vi "Main.vi"() -> ()   [LabVIEW 2020]
doc: "This Continuous Measurement sample project is based on the Queued Message Handler template.\n\nThe Event Handling Loop generates messages based on user interface actions.\n\nThe Message Handling Loop processes messages generated by the Event Handling Loop, or by other messages. There are also Acquisition and Logging message handling loop subVIs, and a chart updating loop."
uses:
  controls/UI Data.ctl
  Modbus/Modbus All Data.ctl
  Modbus/Modbus PLC Data All.ctl
  Modbus/Modbus FVIR Control.ctl
  Modbus/Modbus LDO Control.ctl
  WritingDataFile/Data to Save.ctl
  Modbus/Modbus Gas Meter Data.ctl
  Drivers/Alicat LabVIEW Drivers 2v1/Sub-VIs/Data Cluster.ctl
  Drivers/Alicat LabVIEW Drivers 2v1/Sub-VIs/Units of Measure.ctl
  Drivers/Inficon Transmitter/Type Definitions/Inficon Data.ctl
  support/Event Booleans.ctl
  support/Message Queue/Enqueue Message (Single).vi
  <vilib>/Utility/error.llb/Error Cluster From Error Code.vi
  <vilib>/ErrorRing/Error Ring.xnode
  support/User Event - Stop/User Event - Stop.lvlib
  support/Message Queue/Message Queue.lvlib
  Modbus/Modbus.lvlib
  ReadingDataFile/ReadingDataFile.lvlib
  WritingDataFile/WritingDataFile.lvlib
panel:
  in  "Start Auto GPM Gallons":dbl=5.0 format="%#_13g"
  in  "Debug":bool
  out "Message Loop":string[](array[string])
  out "Event Loop":i32
  out "UI Message Loop":i32
  in  "Tab Control":enum32{"FVIR", "LDO", "Administrator"}(tab)
  out "Actuator spill can is going to Work Pos - FVIR":bool
  out "Actuator spill can is going to Home Pos - FVIR":bool
  out "Actuator mannequin is going to Work Pos - FVIR":bool
  out "Actuator mannequin is going to Home Pos - FVIR":bool
  out "Error - FVIR":bool caption="Error"
  out "Status for error - FVIR":string caption="Error status for FVIR"
  in  "Move mannequin - Go to Work Pos":bool
  in  "Move mannequin - Go to Home Pos":bool
  in  "Spill can - Go to Work Pos":bool
  in  "Spill can - Go to Home Pos":bool
  out "Start recording data - FVIR":bool
  out "Test chamber is in sequence - FVIR":bool
  out "Can is spilling - FVIR":bool
  out "Mannequin is moving - FVIR":bool
  in  "Select test case":i32(listbox)
  in  "Stop Test Case FVIR":bool
  in  "Start Test Case FVIR":bool
  in  "Water Outlet Valve Close FVIR":bool
  in  "Water Outlet Valve Open FVIR":bool
  in  "Gas Solenoid Valve Close FVIR":bool
  in  "Gas Solenoid Valve Open FVIR":bool
  in  "Water Inlet Valve Close FVIR":bool
  in  "Water Inlet Valve Open FVIR":bool
  in  "Water Flow Intellifaucet DRK375 Close FVIR":bool
  in  "Water Flow Intellifaucet DRK375 Open FVIR":bool
  out "Temperatures - FVIR":string[][](array[string])
  out "Sensors - FVIR":string[][](array[string])
  in  "Water Outlet Flow Proportional Valve EPV-312B Close FVIR":bool
  in  "Water Outlet Flow Proportional Valve EPV-312B Open FVIR":bool
  out "Water Outlet Flow Proportional - FVIR":bool
  out "Water flow DRK375 is open - FVIR":bool
  out "Gas Solenoid Valuce - FVIR":bool
  out "Water Inlet Valve - FVIR":bool
  out "Water Outlet Valve - FVIR":bool
  out "General status for FVIR":string
  out "Higher than 1.8% butane":bool
  in  "Start":bool
  in  "Stop":bool
  in  "Path to local logfile":path=path "C:/Users/christian.hansen/Desktop/GE Appliance - FVIR/GEA_Labview_FVIR/CH1234dummy.LOG"
  in  "Reset Flow Meter":bool
  in  "Blower OFF":bool
  in  "Blower ON":bool
  in  "Conveyor OFF":bool
  in  "Conveyor ON":bool
  out "Blower":bool
  out "Conveyor":bool
  in  "Gas Meter Tare Total":bool
  in  "Gas Meter Tare Rate":bool
  out "Data":string[][](array[string])
  in  "Proportioning Valve":dbl(slide) max=100.0 scale=0.0..100.0
  in  "Valve % Open":dbl(slide)=15.0 min=15.0 max=100.0 scale=15.0..100.0
  in  "Temp (°F)":dbl(slide)=32.0 min=32.0 max=203.0 scale=32.0..200.0
  in  "Water Flow Intellifaucet DRK375 Open LDO":bool
  in  "Water Flow Intellifaucet DRK375 Close LDO":bool
  out "Rotary Actuator (ON/OFF)":bool
  out "Oil spray 1.33cc/min":bool
  out "Oil spray 1.1cc/min":bool
  out "Oil spray 0.8cc/min":bool
  out "Burner":bool
  out "Start recording data - LDO":bool
  out "Test chamber is in sequence":bool
  in  "Stop Test Case LDO":bool
  in  "Start Test Case LDO":bool
  in  "Water Outlet Valve Close LDO":bool
  in  "Water Outlet Valve Open LDO":bool
  in  "Water Inlet Valve Close LDO":bool
  in  "Water Inlet Valve Open LDO":bool
  in  "Gas Solenoid Valve Close LDO":bool
  in  "Gas Solenoid Valve Open LDO":bool
  in  "Oil Spray 0.8 cc/min Close":bool
  in  "Oil Spray 0.8 cc/min Open":bool
  in  "Oil Spray 1.1 cc/min Close":bool
  in  "Oil Spray 1.1 cc/min Open":bool
  in  "Oil Spray 1.33 cc/min Close":bool
  in  "Oil Spray 1.33 cc/min Open":bool
  in  "Heater OFF":bool
  in  "Heater ON":bool
  out "Water Outlet Flow Proportional":bool
  out "Intellifaucet Start":bool
  out "Gas Solenoid Valve":bool
  out "Water Inlet Valve":bool
  out "Water Outlet Valve":bool
  in  "Temp (°F) - Automatic Mode":dbl=70.0 min=32.0 max=203.0
  in  "Valve % Open - Automatic Mode":dbl=50.0 min=15.0 max=100.0
  in  "Precondition Purge Gallons":u16=200 caption="Precondition Purge Time (Sec)"
  in  "Pilot Rate (BTU/hr)":dbl=600.0
  out "FVIR PLC lifebit":bool
  out "Labview lifebit":bool
  in  "Send parameters to PLC LDO":bool
  in  "Burner cycle 1 to 10 - Duty cycle ON (default 55 min.)":u16=55 caption="Burner cycle 1 to 10 - Duty cycle ON"
  in  "Burner cycle 1 to 10 - Duty cycle OFF (default 5 min.)":u16=5 caption="Burner cycle 1 to 10 - Duty cycle OFF"
  in  "Burner cycle 11 to 12 - Duty cycle ON (default 235 min.)":u16=235 caption="Burner cycle 11 to 12 - Duty cycle ON"
  in  "Burner cycle 11 to 12 - Duty cycle OFF (default 5 min.)":u16=5 caption="Burner cycle 11 to 12 - Duty cycle OFF"
  in  "Burner cycle 13 to end - Duty cycle ON (default 55 min.)":u16=55 caption="Burner cycle 13 to end - Duty cycle ON"
  in  "Burner cycle 13 to end - Duty cycle OFF (default 5 min.)":u16=5 caption="Burner cycle 13 to end - Duty cycle OFF"
  in  "Oil 1st sequence ON (default 5 min.)":u16=5 caption="Oil 1st sequence ON"
  in  "Oil 1st sequence OFF (default 5 min.)":u16=25 caption="Oil 1st sequence OFF"
  in  "All subsequent sequence ON (default 3 min.)":u16=3 caption="All subsequent sequence ON"
  in  "All subsequent sequence OFF (default 27 min.)":u16=27 caption="All subsequent sequence OFF"
  in  "Oil spray preconditioning period ON (default 10 min.)":u16=10 caption="Oil spray preconditioning period ON"
  in  "Oil spray preconditioning period OFF  (default 20 min.)":u16=20 caption="Oil spray preconditioning period OFF"
  out "General status for LDO":string
  out "Status for error - LDO":string caption="Error status for LDO"
  out "Error - LDO":bool caption="Error"
  in  "PLC IP address":string="10.2.0.11"
  in  "Inficon IP Address":string="192.168.1.32"
  in  "Ultramat 23":refnum<visa-resource-name>="ULTRAMAT"
  in  "Alicat VISA":refnum<visa-resource-name>="ALICAT_40SLPM"
  in  "Send parameters to PLC FVIR":bool
  in  "Time Pause Between Next Mannequin Sequence":u16=60
  in  "Water Flow Intellifaucet DRK375":u16=15
  in  "Water Temperature Intellifaucet DRK375":u16=70
  in  "Water Outlet Proportional Valve EPV-312B":u16=3
  in  "Number of Mannequin Movement":u16=3
  in  "Time Delay of Change direction of Mannequin Actuators":u16=1000
  # "FVIR and LDO:Swap the data, i.e. 28-10-2021 --> 2021-10-28. --> Lets test this first to see the currents PC timeformat. \nAll data is in the file now. Also the status of LEDs and what Labview is sending --> A lot of redundant info here. What from \nLabview --> PLC should be recorded?"
  # "FVIR: Missing implementation: Getting the glas flow rate, SQRH. CO, CO2 and O2 from the VI's from GEA"
  # "FVIR"
  # "Main control"
  # "Actuator spill can is going to Work Pos"
  # "Actuator spill can is going to Home Pos"
  # "Actuator mannequin is going to Work Pos"
  # "Actuator mannequin is going to Home Pos"
  # "Automatic mode"
  # "Start recording FVIR data"
  # "Test chamber is in sequence"
  # "Can is spilling"
  # "Mannequin is moving"
  # "Water Outlet Valve"
  # "Gas Solenoid Valve"
  # "Water Inlet Valve"
  # "Water Flow Intellifaucet DRK375"
  # "Water Outlet Flow Proportional EPV-312B"
  # "Water Outlet Flow Proportional is open"
  # "Water flow DRK375 is open"
  # "Gas Solenoid is open"
  # "Water Inlet is open"
  # "Water Outlet is open"
  # "Status of valves"
  # "Manual mode"
  # "Temperature from textfile - 4 channels"
  # "Status of actuators"
  # "Values from FVIR sensors"
  # "Status of chamber"
  # "Main control"
  # "Manual mode"
  # "Rotary Actuator"
  # "Status of devices"
  # "Status of chamber"
  # "Status of valves"
  # "Water Flow Intellifaucet DRK375"
  # "Water Flow Meter"
  # "Blower Control"
  # "Conveyor Control"
  # "Gas Meter"
  # "Automatic mode"
  # "Start and stop LDO test"
  # "Water Outlet Valve"
  # "Water Inlet Valve"
  # "Gas Solenoid Valve"
  # "Oil spray at 0.8 cc/min"
  # "Oil spray at 1.1 cc/min"
  # "Oil spray at 1.33 cc/min"
  # "LDO Parameters -"
  # "Changing parameters to PLC"
  # "FVIR Changing parameters to PLC"
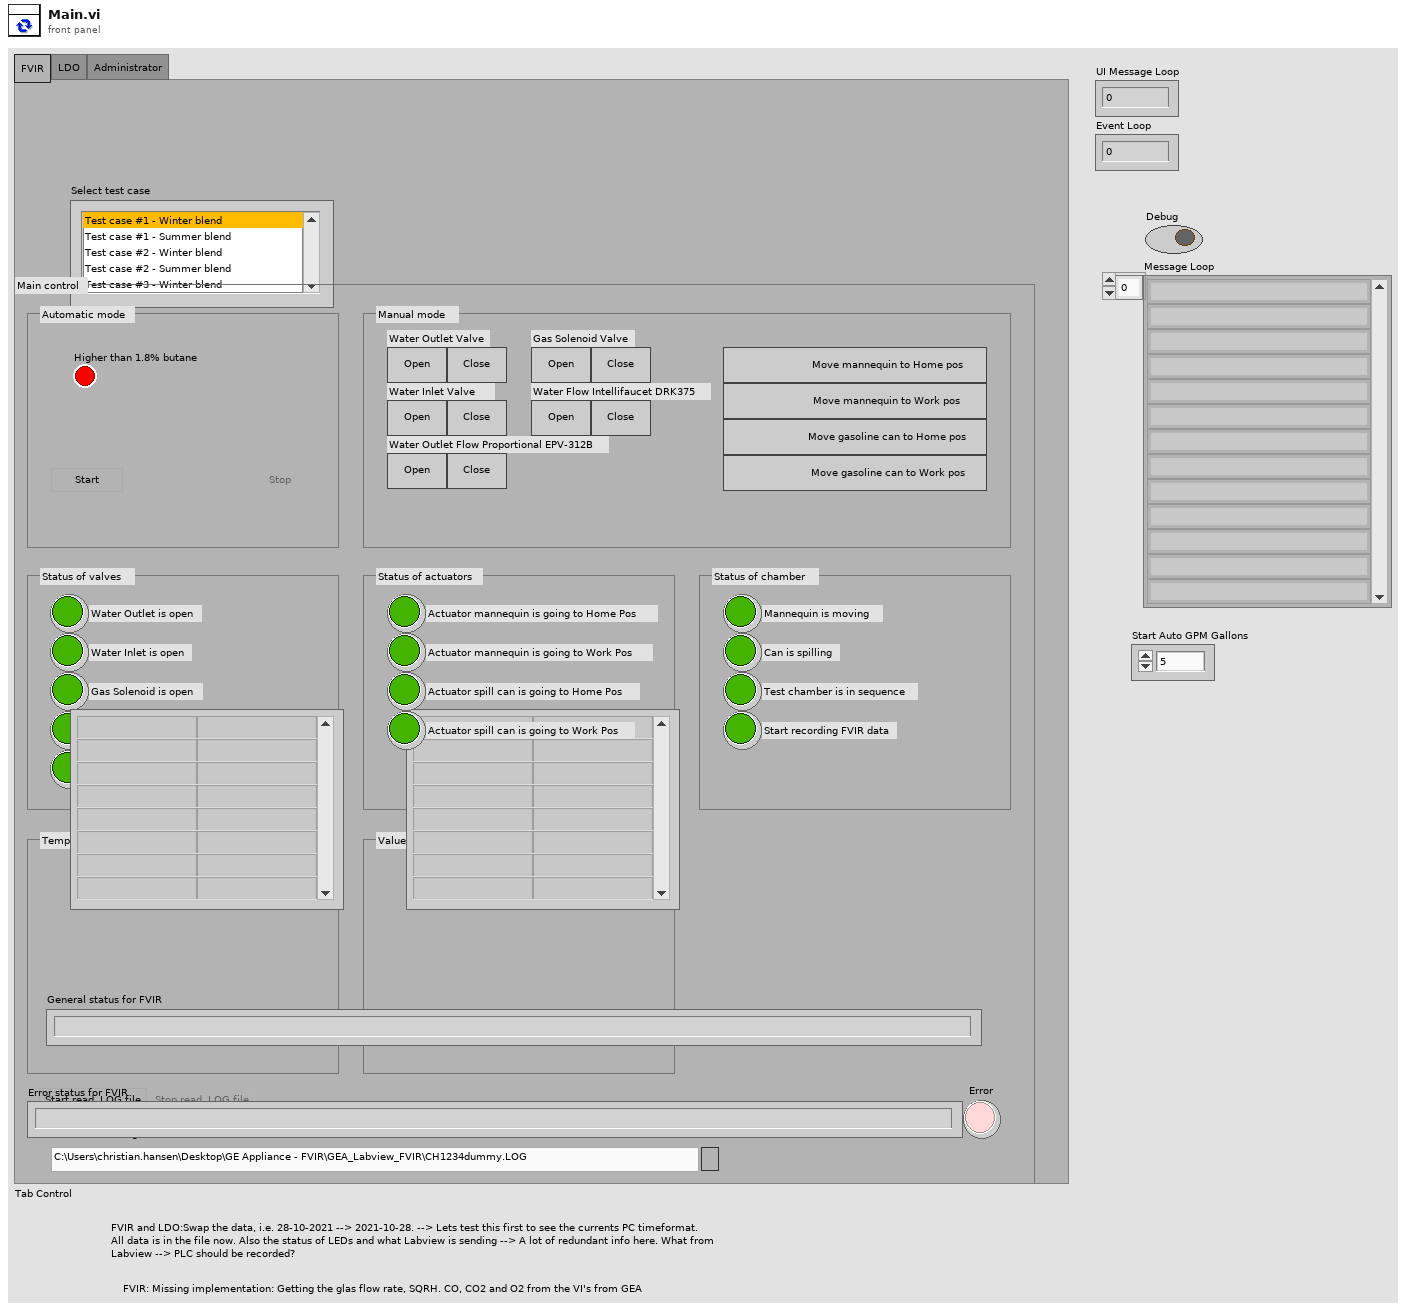
[diagram p1: front panel]
types:
  T1 = typedef "Event Booleans.ctl" = cluster{"Burner ON":bool, "0.8 ml Bool":bool, "1.1 Bool":bool, "1.33 Bool":bool, "Start recording data-LDO":bool}
  T2 = typedef "Modbus All Data.ctl" = cluster{"PLC Data Out":T3, "Gas Data":T7, "Inficon Data Input":T10, "Ultramat 23":string[][]}
  T3 = typedef "Modbus PLC Data All.ctl" = cluster{"FVIR Data Input":T4, "LDO Control Input":T5, "PLC Input Registers":i16[], "Data to Save":T6}
  T4 = typedef "Modbus FVIR Control.ctl" = cluster{"Spare 15":bool, "Spare 14":bool, "Actuator mannequin is going to Work Pos - FVIR":bool, "Actuator mannequin is going to Home Pos - FVIR":bool, "Test chamber is in sequence - FVIR ":bool, "Water flow DRK375 is open - FVIR":bool, "Gas Solenoid Valve - FVIR":bool, "Water Inlet Valve - FVIR":bool, "Water Outlet Flow Proportional - FVIR":bool, "Start recording data - FVIR":bool, "Actuator spill can is going to Work Pos - FVIR":bool, "Actuator spill can is going to Home Pos - FVIR":bool, "Water Outlet Valve - FVIR":bool, "Can is spilling - FVIR":bool, "Mannequin is moving - FVIR":bool, "FVIR PLC lifebit":bool, "Status for Error - FVIR":string, "Error-FVIR":bool, "Sensors -FVIR":string[][]}
  T5 = typedef "Modbus LDO Control.ctl" = cluster{"LDO PLC Life Bit":bool, "Start recording data - LDO":bool, "Spare 1":bool, "Water Outlet Valve - LDO":bool, "Water Inlet Valve - LDO":bool, "Gas Solenoid Valve - LDO":bool, "Water flow DRK375 is open - LDO":bool, "Test chamber is in sequence - LDO":bool, "Oil spray 0.8cc/min - LDO":bool, "Oil spray 1.1cc/min - LDO":bool, "Oil spray 1.33cc/min - LDO":bool, "Rotary Actuator (ON/OFF) - LDO":bool, "Water Outlet Flow Proportional - LDO":bool, "Conveyor ON/OFF":bool, "Blower ON/OFF":bool, "Spare 4":bool, "Status for error - LDO":string, "Error - LDO":bool, "Sensor Data":string[][], "Thermal Efficiency Rate (GPM)":dbl, "Thermal Efficiency":dbl, "Totalized Flow (Gallons)":dbl, "Counter of oil injections 1.33 cc/min":u16, "Counter of burner cycle":u16, "Counter of oil injections 1.1 cc/min":u16, "Counter of oil injections 0.8 cc/min":u16, "Previous Totalizer (Gallons)":dbl, "Gallon Adder Input":dbl}
  T6 = typedef "Data to Save.ctl" = cluster{"LDO Full Data":string[][], "FVIR Full Data":string[][], "Test Case - FVIR":string, "Test Case - LDO":string}
  T7 = typedef "Modbus Gas Meter Data.ctl" = cluster{"Data Cluster":T8, "Units of Measure Input":T9, "Header Array":string[]}
  T8 = typedef "Data Cluster.ctl" = cluster{"Absolute Pressure":dbl, "Gauge/Diff. Pressure":dbl, "Barometric Pressure":dbl, "Temperature":dbl, "Volumetric Flow":dbl, "Mass Flow":dbl, "Setpoint":dbl, "Valve Drive":dbl, "Totalizer":dbl, "[hr]":dbl, "[min]":dbl, "[sec]":dbl, "Totalizer Average Flow":dbl, "Totalizer Peak Flow":dbl, "Gas selected":string}
  T9 = typedef "Units of Measure.ctl" = cluster{"Abs. Pressure":string, "Gauge/Diff. Press.":string, "Barometric Press.":string, "Temperature":string, "Volume":string, "Mass":string, "Setpoint":string, "Valve Drive":string, "Totalizer":string, "Tot. Timer":string, "Tot. Avg. Flow":string, "Tot. Peak Flow":string}
  T10 = typedef "Inficon Data.ctl" = cluster{"Gross Heating Value, Vol (Real, Dry)":dbl, "Nitrogen Component Normalized Mole % (Dry)":dbl, "Methane Component Normalized Mole % (Dry)":dbl, "Carbon Dioxide Component Normalized Mole % (Dry)":dbl, "Ethane Component Normalized Mole % (Dry)":dbl, "Propane Component Normalized Mole % (Dry)":dbl, "i-Pentane Component Normalized Mole % (Dry)":dbl, "i-Butane Component Normalized Mole % (Dry)":dbl, "n-Butane Component Normalized Mole % (Dry)":dbl, "n-Pentane Component Normalized Mole % (Dry)":dbl, "Hexane Component Normalized Mole % (Dry)":dbl, "Heptane Component Normalized Mole % (Dry)":dbl, "Gross Wobbe Index, Real(Dry)":dbl, "Relative Density, Real(Dry)":dbl, "Propylene Component Normalized Mole % (Dry)":dbl, "C4 Olefins Component Normalized Mole % (Dry)":dbl, "Water Component Normalized Mole % (Dry)":dbl}
  T11 = typedef "UI Data.ctl" = cluster{"Start Ref":refnum<vi>, "Stop Ref":refnum<vi>, "Exit Ref":refnum<vi>, "Status Ref":refnum<vi>, "Connect Ref":refnum<vi>, "Disconnect Ref":refnum<vi>, "Spill can Home pos Ref":refnum<vi>, "Spill can Work pos Ref":refnum<vi>, "Move Mannequin Home pos Ref":refnum<vi>, "Move Mannequin Work pos Ref":refnum<vi>, "Start test case FVIR Ref":refnum<vi>, "Water Outlet Valve Open FVIR Ref":refnum<vi>, "Water Inlet Valve Open FVIR Ref":refnum<vi>, "Gas Solenoid Valve Open FVIR Ref":refnum<vi>, "Water Flow Open FVIR Ref":refnum<vi>, "Listbox Ref":refnum<vi>, "Stop test case FVIR Ref":refnum<vi>, "Water Outlet Valve Close FVIR Ref":refnum<vi>, "Water Inlet Valve Close FVIR Ref":refnum<vi>, "Gas Solenoid Valve Close FVIR Ref":refnum<vi>, "Water Flow Close FVIR Ref":refnum<vi>, "Send Param to PLC FVIR Ref":refnum<vi>, "Water Flow Prop Open FVIR Ref":refnum<vi>, "Water Flow Prop Close FVIR Ref":refnum<vi>, "Start test case LDO Ref":refnum<vi>, "Stop test case LDO Ref":refnum<vi>, "Water Outlet Valve Open LDO Ref":refnum<vi>, "Water Outlet Valve Close LDO Ref":refnum<vi>, "Water Inlet Valve Open LDO Ref":refnum<vi>, "Water Inlet Valve Close LDO Ref":refnum<vi>, "Gas Solenoid Valve Open LDO Ref":refnum<vi>, "Gas Solenoid Valve Close LDO Ref":refnum<vi>, "Water Flow Open LDO Ref":refnum<vi>, "Water Flow Close LDO Ref":refnum<vi>, "Water Flow Prop Open LDO Ref":refnum<vi>, "Water Flow Prop Close LDO Ref":refnum<vi>, "Oil spray 0.8cc/min Open Ref":refnum<vi>, "Oil spray 0.8cc/min Close Ref":refnum<vi>, "Oil spray 1.1cc/min Open Ref":refnum<vi>, "Oil spray 1.1cc/min Close Ref":refnum<vi>, "Oil spray 1.33cc/min Open Ref":refnum<vi>, "Oil spray 1.33cc/min Close Ref":refnum<vi>, "Heater ON Ref":refnum<vi>, "Heater OFF Ref":refnum<vi>, "Send Param to PLC LDO Ref":refnum<vi>}
  T12 = typedef "Message Queue.lvlib/All Message Queues.ctl" = cluster{"UI":refnum<queue>, "Modbus":refnum<queue>, "Watchdog":refnum<queue>, "ReadDataFile":refnum<queue>, "DataScanning":refnum<queue>, "WriteDataFile":refnum<queue>, "WatchdogWriteFile":refnum<queue>, "OilMachine":refnum<queue>, "Alicat_GasMeter":refnum<queue>, "Inficon":refnum<queue>, "Ultramat 23":refnum<queue>}
  T13 = enum8{"Enabled", "Disabled", "Disabled and Grayed Out"}
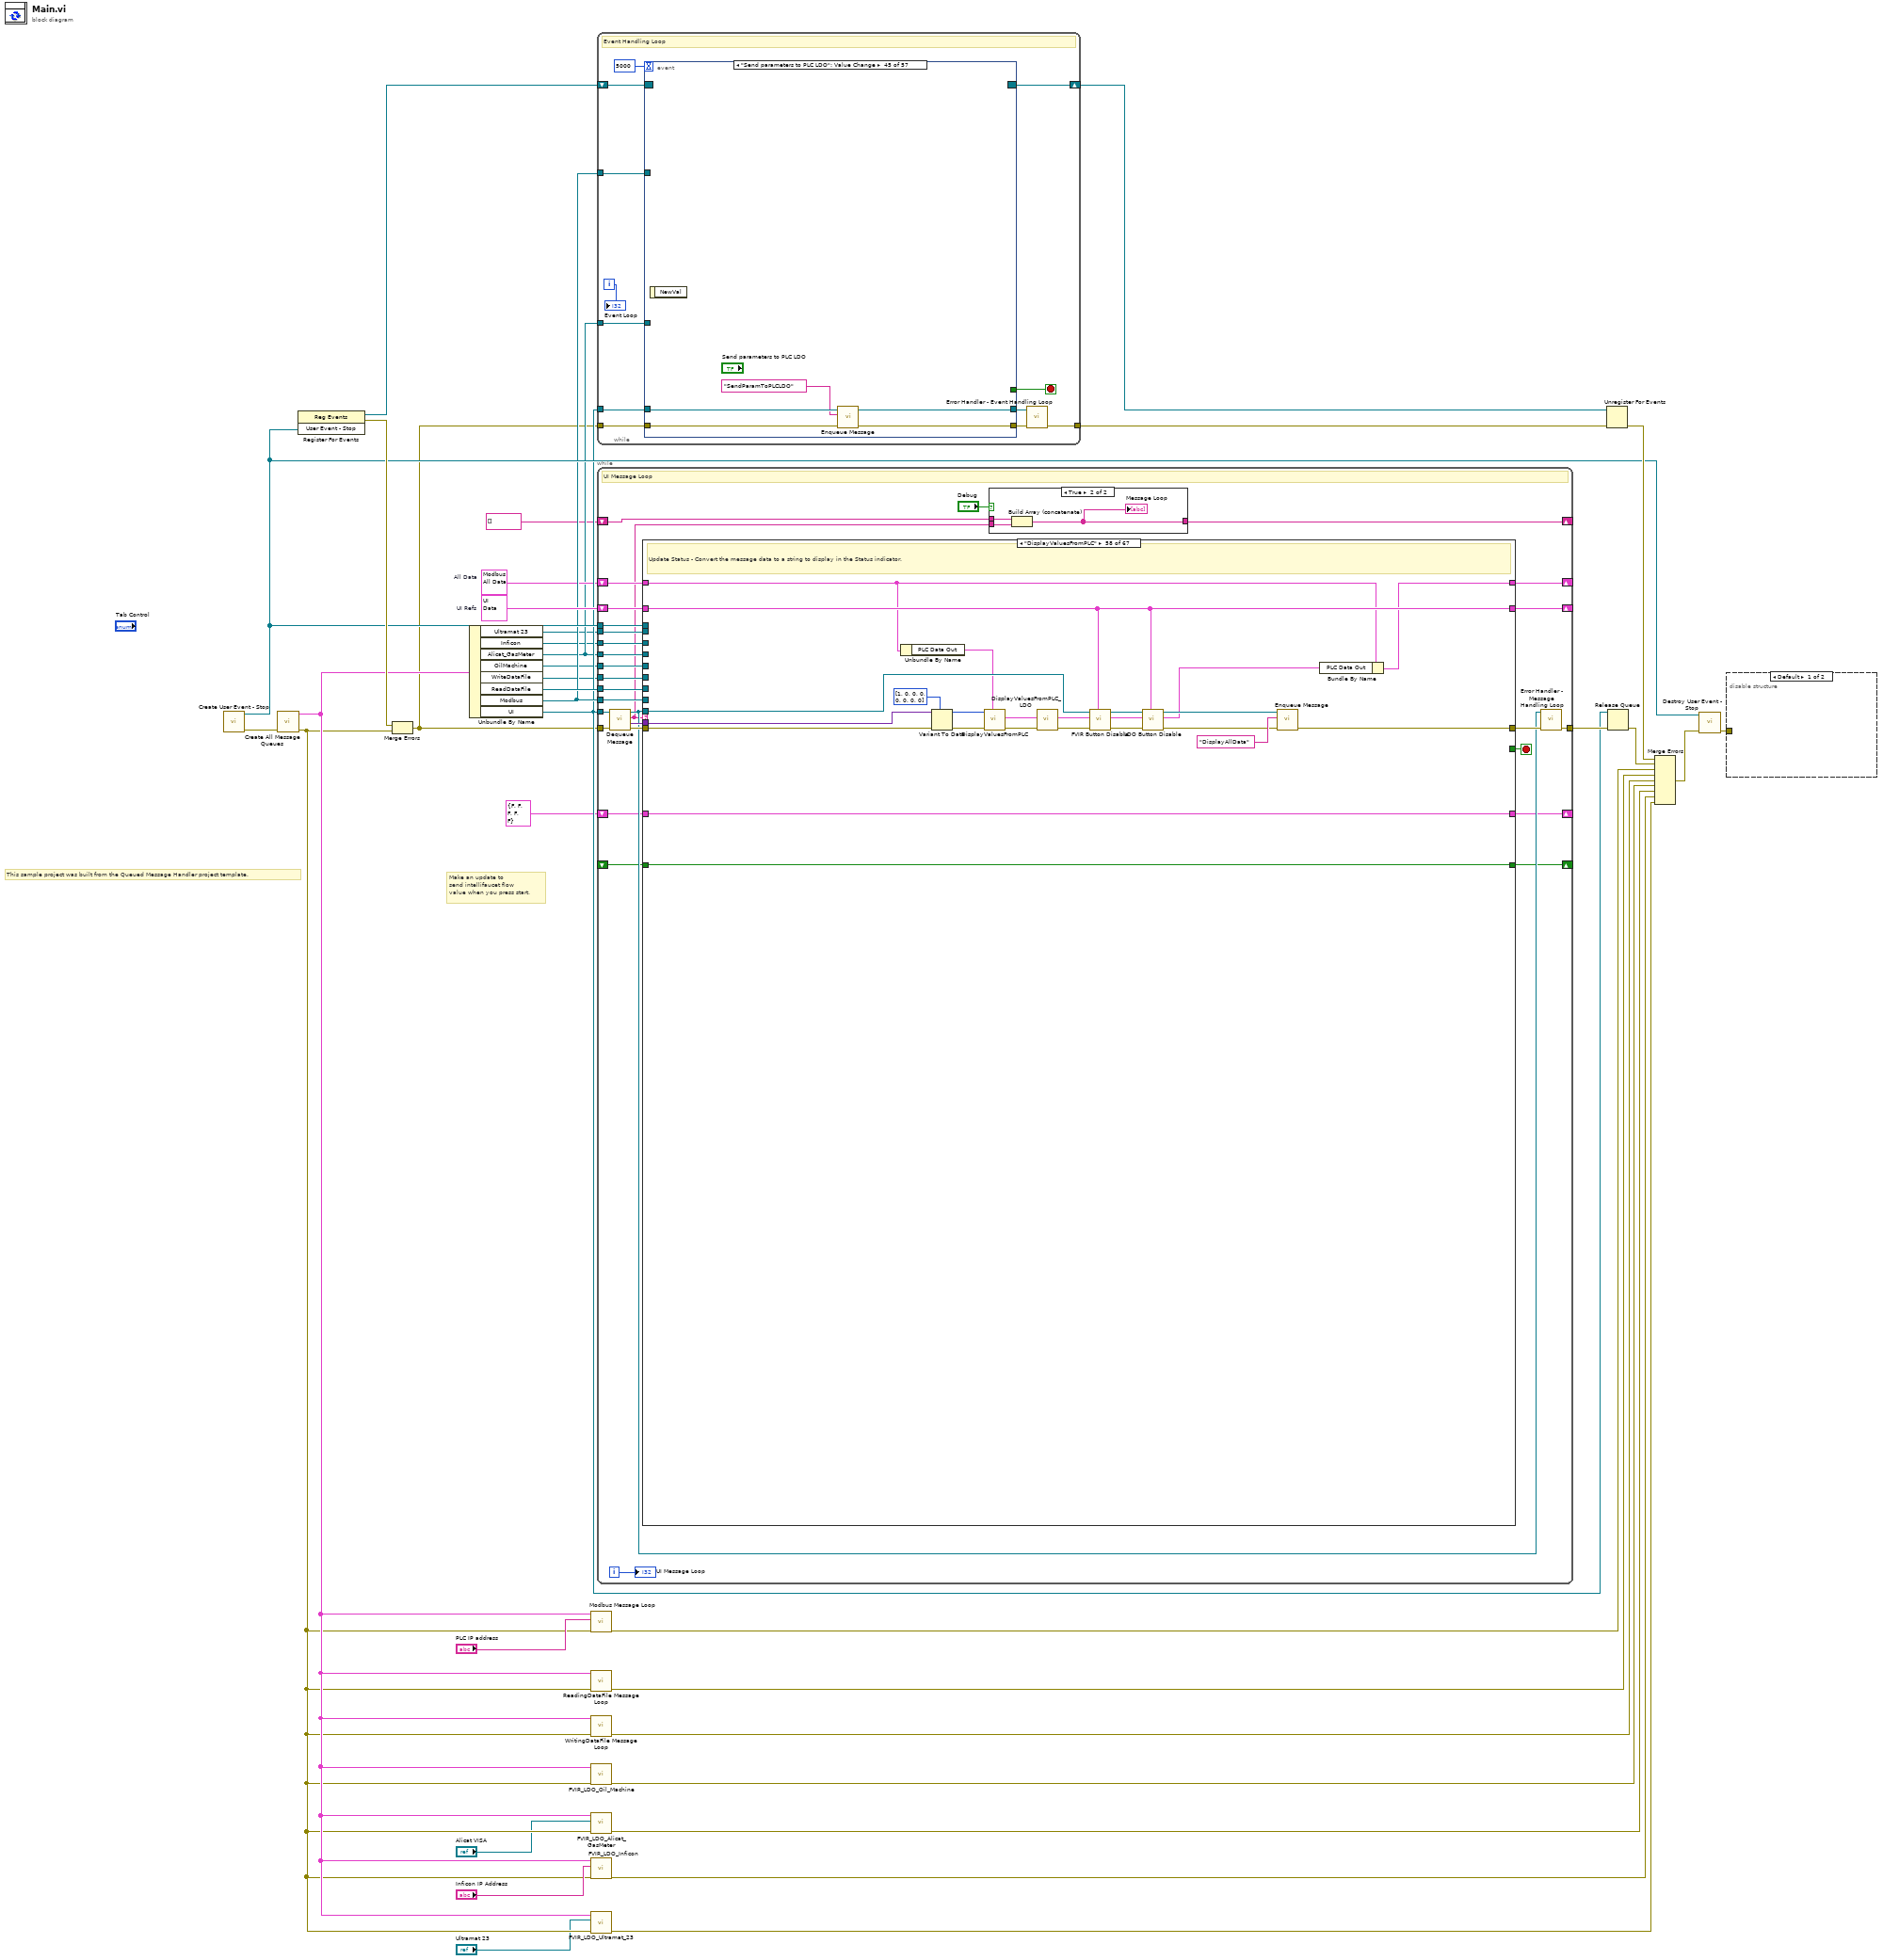
[diagram p0: block diagram]
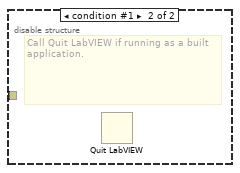
[diagram p2: hidden frame]
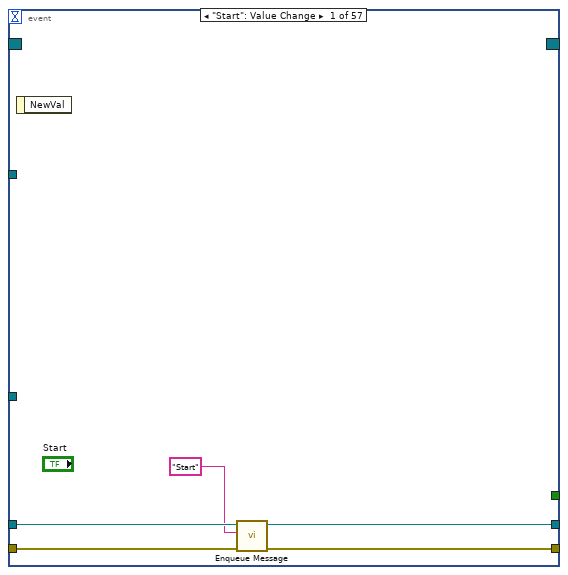
[diagram p3: hidden frame]
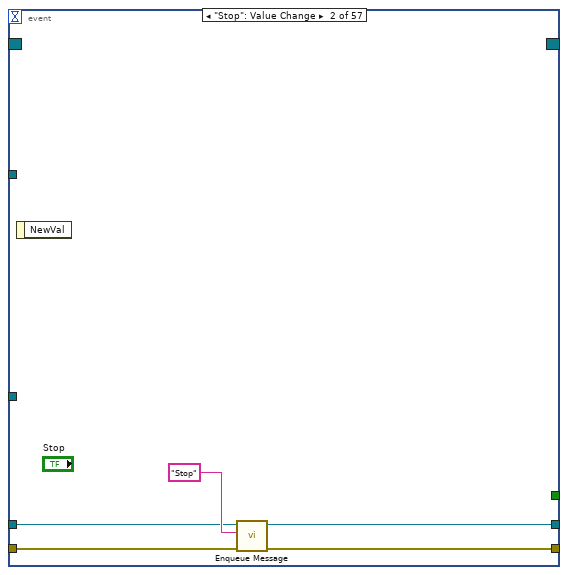
[diagram p4: hidden frame]
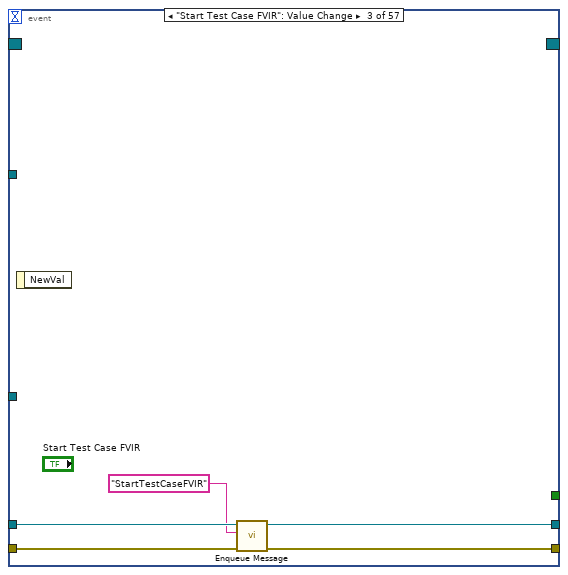
[diagram p5: hidden frame]
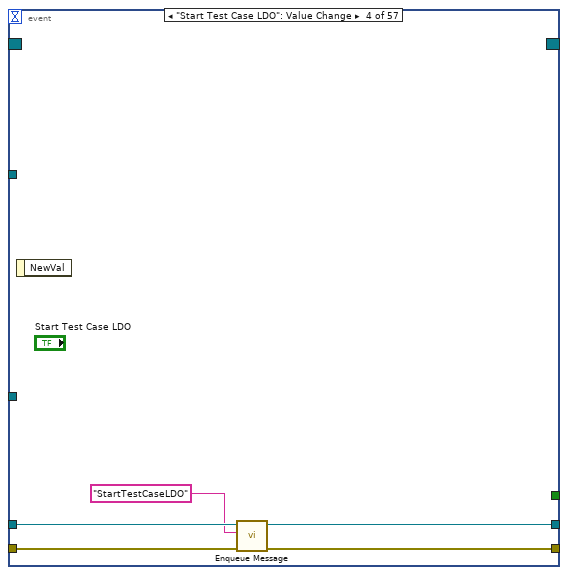
[diagram p6: hidden frame]
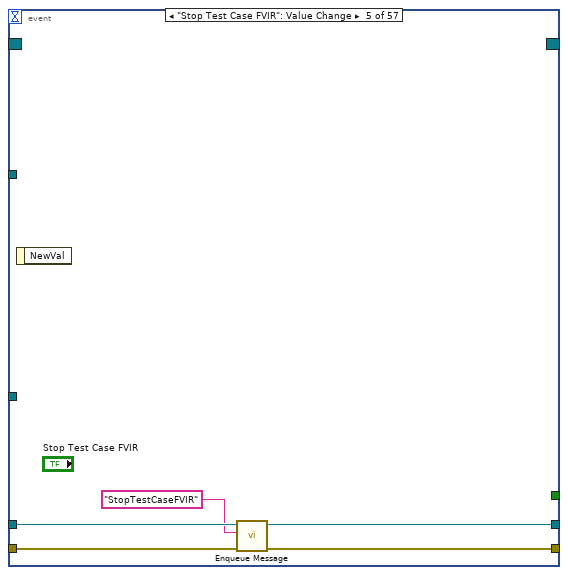
[diagram p7: hidden frame]
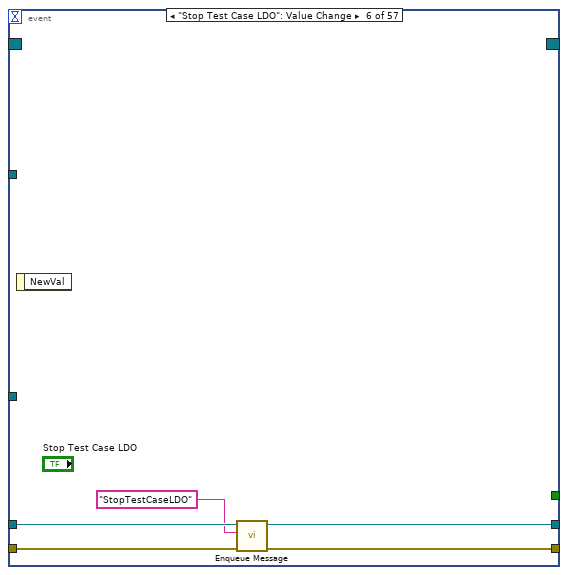
[diagram p8: hidden frame]
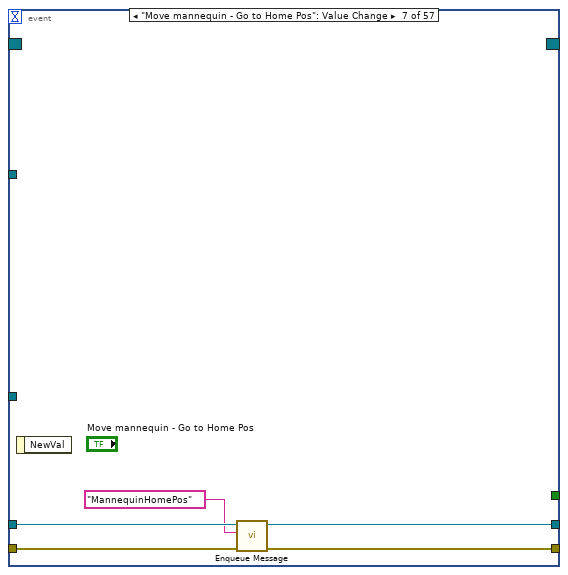
[diagram p9: hidden frame]
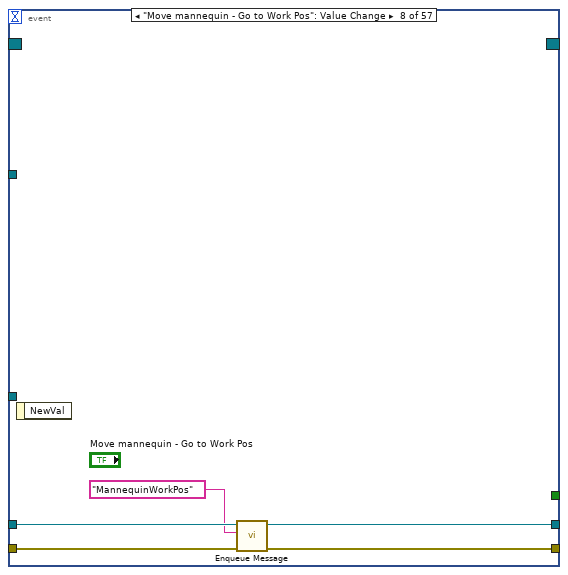
[diagram p10: hidden frame]
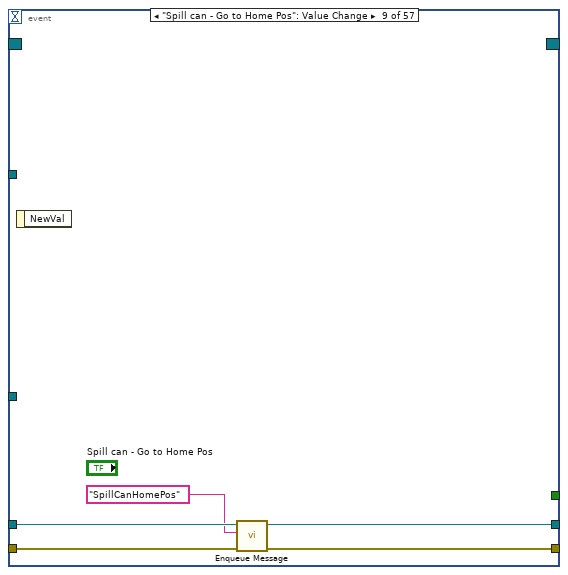
[diagram p11: hidden frame]
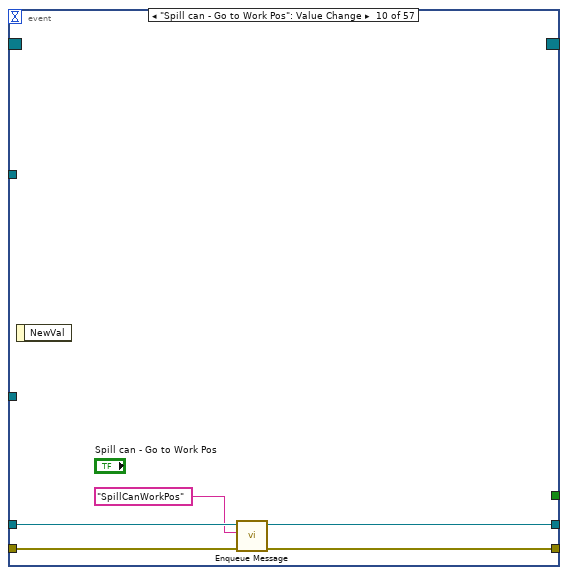
[diagram p12: hidden frame]
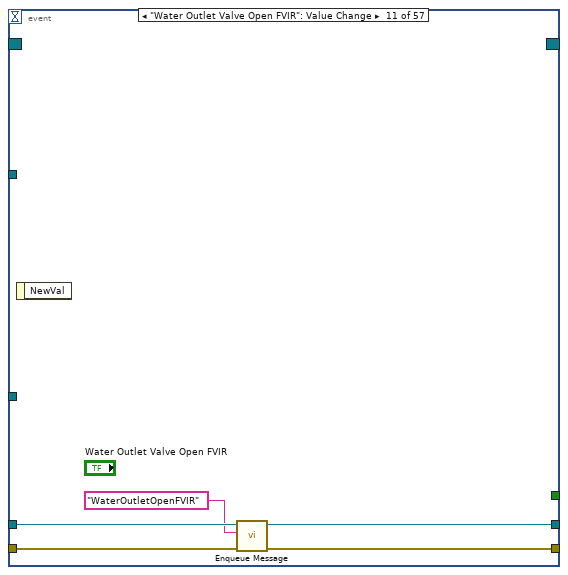
[diagram p13: hidden frame]
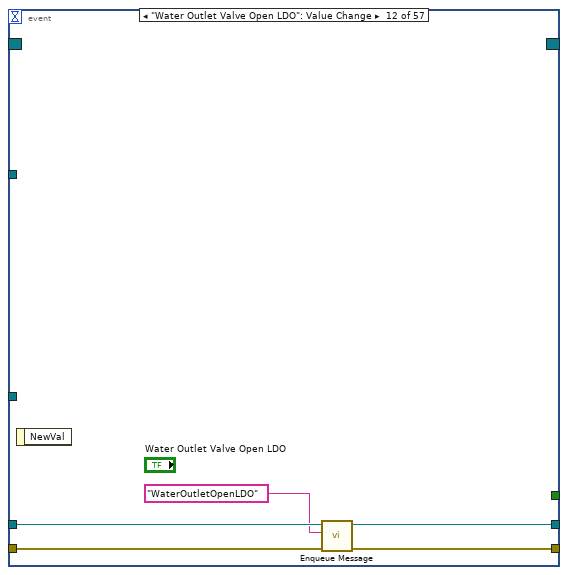
[diagram p14: hidden frame]
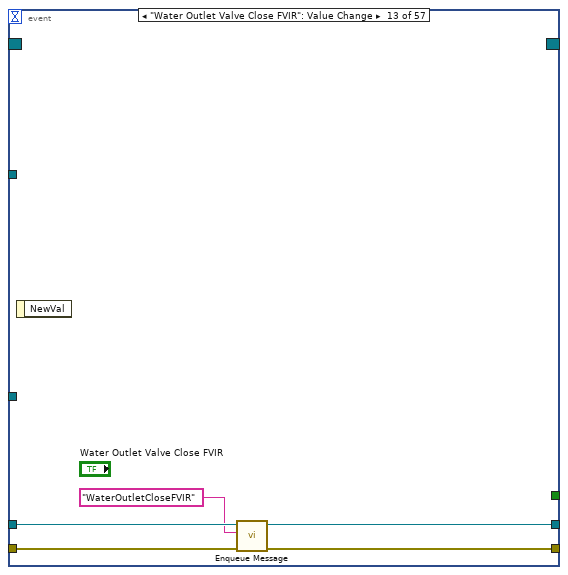
[diagram p15: hidden frame]
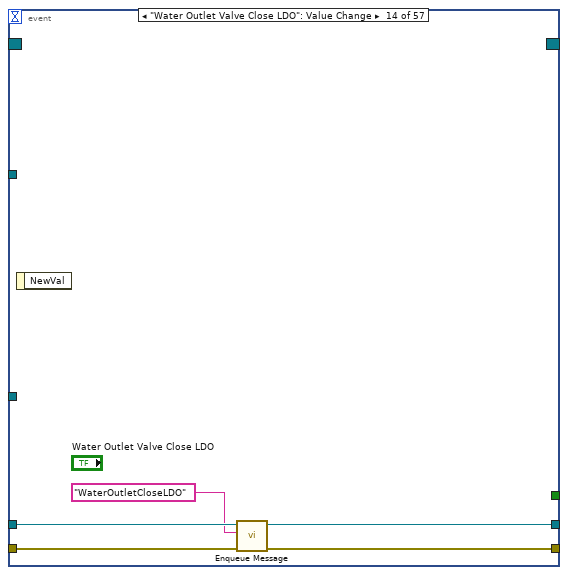
[diagram p16: hidden frame]
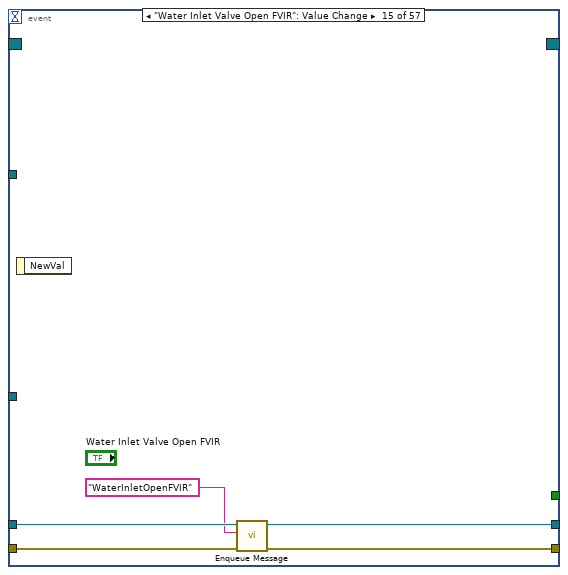
[diagram p17: hidden frame]
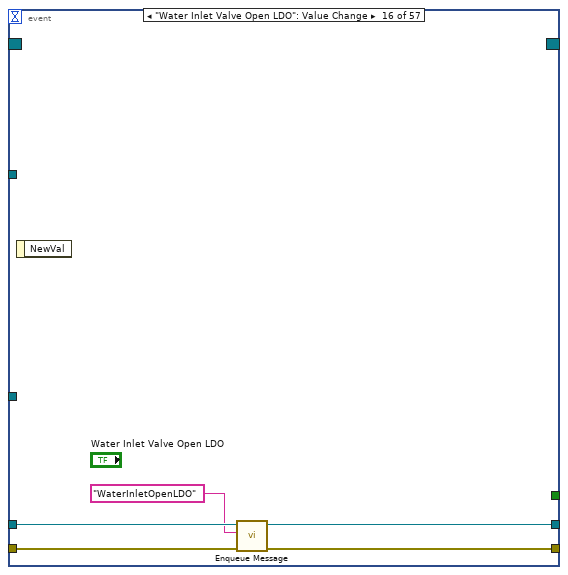
[diagram p18: hidden frame]
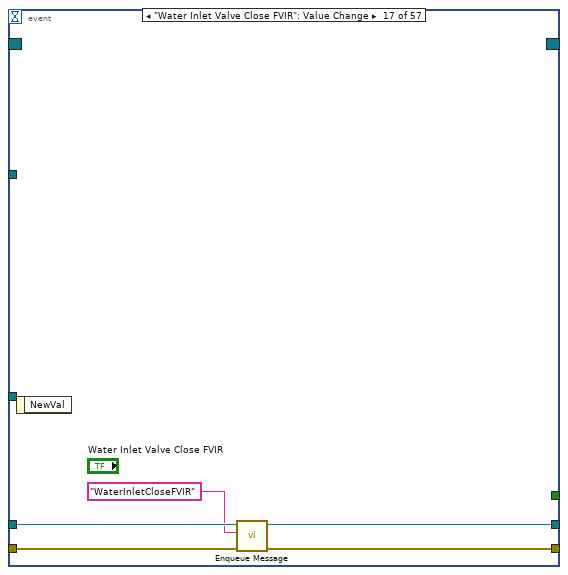
[diagram p19: hidden frame]
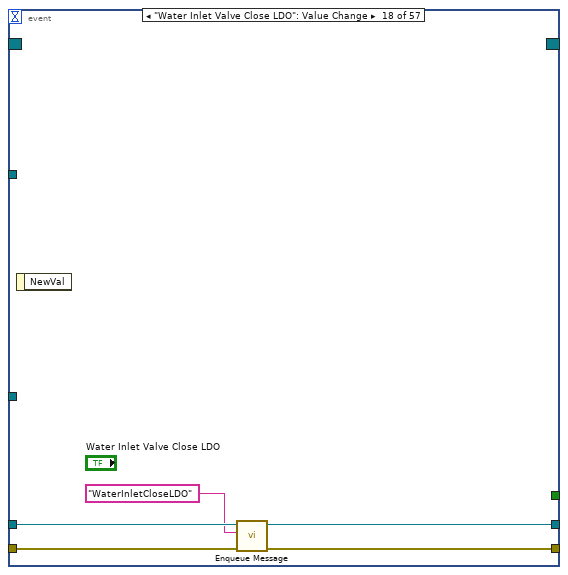
[diagram p20: hidden frame]
diagram:
  w16 = T2 {"PLC Data Out"={"FVIR Data Input"={"Spare 15"=FALSE, "Spare 14"=FALSE, "Actuator mannequin is going to Work Pos - FVIR"=FALSE, "Actuator mannequin is going to Home Pos - FVIR"=FALSE, "Test chamber is in sequence - FVIR "=FALSE, "Water flow DRK375 is open - FVIR"=FALSE, "Gas Solenoid Valve - FVIR"=FALSE, "Water Inlet Valve - FVIR"=FALSE, "Water Outlet Flow Proportional - FVIR"=FALSE, "Start recording data - FVIR"=FALSE, "Actuator spill can is going to Work Pos - FVIR"=FALSE, "Actuator spill can is going to Home Pos - FVIR"=FALSE, "Water Outlet Valve - FVIR"=FALSE, "Can is spilling - FVIR"=FALSE, "Mannequin is moving - FVIR"=FALSE, "FVIR PLC lifebit"=FALSE, "Status for Error - FVIR"="", "Error-FVIR"=FALSE, "Sensors -FVIR"=[]}, "LDO Control Input"={"LDO PLC Life Bit"=FALSE, "Start recording data - LDO"=FALSE, "Spare 1"=FALSE, "Water Outlet Valve - LDO"=FALSE, "Water Inlet Valve - LDO"=FALSE, "Gas Solenoid Valve - LDO"=FALSE, "Water flow DRK375 is open - LDO"=FALSE, "Test chamber is in sequence - LDO"=FALSE, "Oil spray 0.8cc/min - LDO"=FALSE, "Oil spray 1.1cc/min - LDO"=FALSE, "Oil spray 1.33cc/min - LDO"=FALSE, "Rotary Actuator (ON/OFF) - LDO"=FALSE, "Water Outlet Flow Proportional - LDO"=FALSE, "Conveyor ON/OFF"=FALSE, "Blower ON/OFF"=FALSE, "Spare 4"=FALSE, "Status for error - LDO"="", "Error - LDO"=FALSE, "Sensor Data"=[], "Thermal Efficiency Rate (GPM)"=0.0, "Thermal Efficiency"=0.0, "Totalized Flow (Gallons)"=0.0, "Counter of oil injections 1.33 cc/min"=0, "Counter of burner cycle"=0, "Counter of oil injections 1.1 cc/min"=0, "Counter of oil injections 0.8 cc/min"=0, "Previous Totalizer (Gallons)"=0.0, "Gallon Adder Input"=0.0}, "PLC Input Registers"=[], "Data to Save"={"LDO Full Data"=[], "FVIR Full Data"=[], "Test Case - FVIR"="", "Test Case - LDO"=""}}, "Gas Data"={"Data Cluster"={"Absolute Pressure"=0.0, "Gauge/Diff. Pressure"=0.0, "Barometric Pressure"=0.0, "Temperature"=0.0, "Volumetric Flow"=0.0, "Mass Flow"=0.0, "Setpoint"=0.0, "Valve Drive"=0.0, "Totalizer"=0.0, "[hr]"=0.0, "[min]"=0.0, "[sec]"=0.0, "Totalizer Average Flow"=0.0, "Totalizer Peak Flow"=0.0, "Gas selected"=""}, "Units of Measure Input"={"Abs. Pressure"="", "Gauge/Diff. Press."="", "Barometric Press."="", "Temperature"="", "Volume"="", "Mass"="", "Setpoint"="", "Valve Drive"="", "Totalizer"="", "Tot. Timer"="", "Tot. Avg. Flow"="", "Tot. Peak Flow"=""}, "Header Array"=[]}, "Inficon Data Input"={"Gross Heating Value, Vol (Real, Dry)"=0.0, "Nitrogen Component Normalized Mole % (Dry)"=0.0, "Methane Component Normalized Mole % (Dry)"=0.0, "Carbon Dioxide Component Normalized Mole % (Dry)"=0.0, "Ethane Component Normalized Mole % (Dry)"=0.0, "Propane Component Normalized Mole % (Dry)"=0.0, "i-Pentane Component Normalized Mole % (Dry)"=0.0, "i-Butane Component Normalized Mole % (Dry)"=0.0, "n-Butane Component Normalized Mole % (Dry)"=0.0, "n-Pentane Component Normalized Mole % (Dry)"=0.0, "Hexane Component Normalized Mole % (Dry)"=0.0, "Heptane Component Normalized Mole % (Dry)"=0.0, "Gross Wobbe Index, Real(Dry)"=0.0, "Relative Density, Real(Dry)"=0.0, "Propylene Component Normalized Mole % (Dry)"=0.0, "C4 Olefins Component Normalized Mole % (Dry)"=0.0, "Water Component Normalized Mole % (Dry)"=0.0}, "Ultramat 23"=[]}  # All Data
  w32 = T11 {"Start Ref"=refnum, "Stop Ref"=refnum, "Exit Ref"=refnum, "Status Ref"=refnum, "Connect Ref"=refnum, "Disconnect Ref"=refnum, "Spill can Home pos Ref"=refnum, "Spill can Work pos Ref"=refnum, "Move Mannequin Home pos Ref"=refnum, "Move Mannequin Work pos Ref"=refnum, "Start test case FVIR Ref"=refnum, "Water Outlet Valve Open FVIR Ref"=refnum, "Water Inlet Valve Open FVIR Ref"=refnum, "Gas Solenoid Valve Open FVIR Ref"=refnum, "Water Flow Open FVIR Ref"=refnum, "Listbox Ref"=refnum, "Stop test case FVIR Ref"=refnum, "Water Outlet Valve Close FVIR Ref"=refnum, "Water Inlet Valve Close FVIR Ref"=refnum, "Gas Solenoid Valve Close FVIR Ref"=refnum, "Water Flow Close FVIR Ref"=refnum, "Send Param to PLC FVIR Ref"=refnum, "Water Flow Prop Open FVIR Ref"=refnum, "Water Flow Prop Close FVIR Ref"=refnum, "Start test case LDO Ref"=refnum, "Stop test case LDO Ref"=refnum, "Water Outlet Valve Open LDO Ref"=refnum, "Water Outlet Valve Close LDO Ref"=refnum, "Water Inlet Valve Open LDO Ref"=refnum, "Water Inlet Valve Close LDO Ref"=refnum, "Gas Solenoid Valve Open LDO Ref"=refnum, "Gas Solenoid Valve Close LDO Ref"=refnum, "Water Flow Open LDO Ref"=refnum, "Water Flow Close LDO Ref"=refnum, "Water Flow Prop Open LDO Ref"=refnum, "Water Flow Prop Close LDO Ref"=refnum, "Oil spray 0.8cc/min Open Ref"=refnum, "Oil spray 0.8cc/min Close Ref"=refnum, "Oil spray 1.1cc/min Open Ref"=refnum, "Oil spray 1.1cc/min Close Ref"=refnum, "Oil spray 1.33cc/min Open Ref"=refnum, "Oil spray 1.33cc/min Close Ref"=refnum, "Heater ON Ref"=refnum, "Heater OFF Ref"=refnum, "Send Param to PLC LDO Ref"=refnum}  # UI Refs
  # "Make an update to \nsend intellifaucet flow \nvalue when you press start."
  # "This sample project was built from the Queued Message Handler project template."
  n1 = call "Create User Event - Stop.vi"() -> ("error out"=w35:errorcluster, "User Event - Stop"=w27:refnum<user-event>)  [unwired: 10 in]
  n2 = call "Create All Message Queues.vi"("error in (no error)"=w35) -> ("error out"=w11:errorcluster, "Message Queues out"=w12:T12)  [unwired: 9 in]
  n3 = register-events(w27) -> (reference out=w29:refnum<event-registration>, error out=w28:errorcluster)  [unwired: 2 in]
  n4 = Merge Errors(w28, w11) -> (w3:errorcluster)
  n5 = Unbundle By Name(w12) -> ("Ultramat 23"=w6:refnum<queue>, "Inficon"=w14:refnum<queue>, "Alicat_GasMeter"=w15:refnum<queue>, "OilMachine"=w18:refnum<queue>, "WriteDataFile"=w2:refnum<queue>, "ReadDataFile"=w26:refnum<queue>, "Modbus"=w25:refnum<queue>, "UI"=w20:refnum<queue>)
  n6 = call "Modbus Message Loop.vi"("Message Queues in"=w12, "PLC IP address"="PLC IP address", "error in (no error)"=w11) -> ("error out"=w24:errorcluster)  [unwired: 7 in]
  n7 = call "ReadingDataFile Message Loop.vi"("error in (no error)"=w11, "Message Queues"=w12) -> ("error out"=w23:errorcluster)  [unwired: 7 in, 1 out]
  n8 = call "WritingDataFile Message Loop.vi"("error in (no error)"=w11, "Message Queues"=w12) -> ("error out"=w22:errorcluster)  [unwired: 9 in]
  n9 = call "FVIR_LDO_Oil_Machine.vi"("error in"=w11, "Message Queues"=w12) -> ("error out"=w19:errorcluster)  [unwired: 9 in]
  n10 = call "FVIR_LDO_Alicat_GasMeter.vi"("error in"=w11, "VISA Refnum in"="Alicat VISA", "Message Queues"=w12) -> ("error out"=w10:errorcluster)  [unwired: 8 in]
  n11 = call "FVIR_LDO_Inficon.vi"("error in"=w11, "Remote IP Address"="Inficon IP Address", "Message Queues"=w12) -> ("error out"=w9:errorcluster)  [unwired: 8 in]
  n12 = call "FVIR_LDO_Ultramat_23.vi"("error in"=w11, "VISA resource name"="Ultramat 23", "Message Queues"=w12) -> ("error out"=w8:errorcluster)  [unwired: 8 in]
  n13 = while {
    tunnel: w20 -> [w48]
    tunnel: [w45] -> w36
    shift-right: [w47] -> w33
    shift-left: w29 -> [w49]
    tunnel: w25 -> [w41]
    tunnel: w15 -> [w40]
    tunnel: w3 -> [w38]
    i -> [w39]
    stop <- w46 stop-if-true
    # "Event Handling Loop"
    n14 = event shown="[44] \"Send parameters to PLC LDO\": Value Change" {
      selector: w49 -> [_ _ _ _ _ _ _ _ _ _ _ _ _ _ _ _ _ _ _ _ _ _ _ _ _ _ _ _ _ _ _ _ _ _ _ _ _ _ _ _ _ _ _ _ _ _ _ _ _ _ _ _ _ _ _ _ _]
      dyn-events: [_ _ _ _ _ _ _ _ _ _ _ _ _ _ _ _ _ _ _ _ _ _ _ _ _ _ _ _ _ _ _ _ _ _ _ _ _ _ _ _ _ _ _ _ _ _ _ _ _ _ _ _ _ _ _ _ _] -> w47
      timeout: 5000 -> [_ _ _ _ _ _ _ _ _ _ _ _ _ _ _ _ _ _ _ _ _ _ _ _ _ _ _ _ _ _ _ _ _ _ _ _ _ _ _ _ _ _ _ _ _ _ _ _ _ _ _ _ _ _ _ _ _]
      tunnel: [_ _ _ _ _ _ _ _ _ _ _ _ _ _ _ _ _ _ _ _ _ _ _ _ _ _ _ _ _ _ _ _ _ _ _ _ _ _ _ _ _ _ _ _ _ _ _ TRUE ("Discard?") _ _ _ _ _ _ _ _ _] -> w46
      tunnel: w48 -> [w54 w58 w64 w69 w74 w79 w84 w89 w94 w99 w104 w109 w114 w119 w124 w129 w134 w139 w144 w149 w154 w159 w164 w174 w181 w191 w198 w203 w208 w213 w218 w226 w231 w236 w244 w249 w254 w262 w267 w269 w274 w279 w284 w292 w297 w303 w307 w310 w313 w330 w335 w340 w344 w348 w351 w356 w363]
      tunnel: [w52 w57 w62 w67 w72 w77 w82 w87 w92 w97 w102 w107 w112 w117 w122 w127 w132 w137 w142 w147 w152 w157 w162 w170 w179 w189 w196 w201 w206 w211 w217 w224 w229 w234 w242 w247 w252 w260 w265 w270 w275 w280 w285 w290 w295 w301 w306 w308 w318 w326 w331 w336 w341 w345 w349 w354 w361] -> w44
      tunnel: [w51 w56 w61 w66 w71 w76 w81 w86 w91 w96 w101 w106 w111 w116 w121 w126 w131 w136 w141 w146 w151 w156 w161 w171 w178 w187 w195 w200 w205 w210 w216 w223 w228 w235 w241 w246 w253 w259 w264 w268 w273 w278 w283 w289 w294 w302 w307 w310 w312 w330 w335 w340 w344 w348 w351 w356 w363] -> w43
      tunnel: w41 -> [_ _ _ _ _ _ _ _ _ _ _ _ _ _ _ _ _ _ _ _ _ _ _ _ _ _ _ _ _ _ _ _ _ _ _ _ _ _ _ _ _ _ _ _ _ _ _ _ _ w328 w333 w338 _ _ w350 w353 _]
      tunnel: w40 -> [_ _ _ _ _ _ _ _ _ _ _ _ _ _ _ _ _ _ _ _ _ _ _ _ _ _ _ _ _ _ _ _ _ _ _ _ _ _ _ _ _ _ _ _ _ _ _ _ _ _ _ _ w342 w346 _ _ w362]
      tunnel: w38 -> [w50 w55 w60 w65 w70 w75 w80 w85 w90 w95 w100 w105 w110 w115 w120 w125 w130 w135 w140 w145 w150 w155 w160 w165 w177 w182 w194 w199 w204 w209 w214 w222 w227 w232 w240 w245 w250 w258 w263 w271 w276 w281 w286 w288 w293 w299 w306 w308 w317 _ _ _ _ _ _ _ w359]
      event "Start": Value Change {
        n15 = event-data() -> ()  [unwired: 1 in, 1 out]
        n16 = call-poly "Enqueue Message.vi"("error in (no error)"=w50, "Message"="Start", "Message Queue"=w54) -> ("error out"=w52:errorcluster, "dup Message Queue"=w51:refnum<queue>)  [unwired: 7 in]
      }
      event "Stop": Value Change {
        n17 = event-data() -> ()  [unwired: 1 in, 1 out]
        n18 = call-poly "Enqueue Message.vi"("error in (no error)"=w55, "Message"="Stop", "Message Queue"=w58) -> ("error out"=w57:errorcluster, "dup Message Queue"=w56:refnum<queue>)  [unwired: 7 in]
      }
      event "Start Test Case FVIR": Value Change {
        n19 = event-data() -> ()  [unwired: 1 in, 1 out]
        n20 = call-poly "Enqueue Message.vi"("error in (no error)"=w60, "Message"="StartTestCaseFVIR", "Message Queue"=w64) -> ("error out"=w62:errorcluster, "dup Message Queue"=w61:refnum<queue>)  [unwired: 7 in]
      }
      event "Start Test Case LDO": Value Change {
        n21 = event-data() -> ()  [unwired: 1 in, 1 out]
        n22 = call-poly "Enqueue Message.vi"("error in (no error)"=w65, "Message"="StartTestCaseLDO", "Message Queue"=w69) -> ("error out"=w67:errorcluster, "dup Message Queue"=w66:refnum<queue>)  [unwired: 7 in]
      }
      event "Stop Test Case FVIR": Value Change {
        n23 = event-data() -> ()  [unwired: 1 in, 1 out]
        n24 = call-poly "Enqueue Message.vi"("error in (no error)"=w70, "Message"="StopTestCaseFVIR", "Message Queue"=w74) -> ("error out"=w72:errorcluster, "dup Message Queue"=w71:refnum<queue>)  [unwired: 7 in]
      }
      event "Stop Test Case LDO": Value Change {
        n25 = event-data() -> ()  [unwired: 1 in, 1 out]
        n26 = call-poly "Enqueue Message.vi"("error in (no error)"=w75, "Message"="StopTestCaseLDO", "Message Queue"=w79) -> ("error out"=w77:errorcluster, "dup Message Queue"=w76:refnum<queue>)  [unwired: 7 in]
      }
      event "Move mannequin - Go to Home Pos": Value Change {
        n27 = event-data() -> ()  [unwired: 1 in, 1 out]
        n28 = call-poly "Enqueue Message.vi"("error in (no error)"=w80, "Message"="MannequinHomePos", "Message Queue"=w84) -> ("error out"=w82:errorcluster, "dup Message Queue"=w81:refnum<queue>)  [unwired: 7 in]
      }
      event "Move mannequin - Go to Work Pos": Value Change {
        n29 = event-data() -> ()  [unwired: 1 in, 1 out]
        n30 = call-poly "Enqueue Message.vi"("error in (no error)"=w85, "Message"="MannequinWorkPos", "Message Queue"=w89) -> ("error out"=w87:errorcluster, "dup Message Queue"=w86:refnum<queue>)  [unwired: 7 in]
      }
      event "Spill can - Go to Home Pos": Value Change {
        n31 = event-data() -> ()  [unwired: 1 in, 1 out]
        n32 = call-poly "Enqueue Message.vi"("error in (no error)"=w90, "Message"="SpillCanHomePos", "Message Queue"=w94) -> ("error out"=w92:errorcluster, "dup Message Queue"=w91:refnum<queue>)  [unwired: 7 in]
      }
      event "Spill can - Go to Work Pos": Value Change {
        n33 = event-data() -> ()  [unwired: 1 in, 1 out]
        n34 = call-poly "Enqueue Message.vi"("error in (no error)"=w95, "Message"="SpillCanWorkPos", "Message Queue"=w99) -> ("error out"=w97:errorcluster, "dup Message Queue"=w96:refnum<queue>)  [unwired: 7 in]
      }
      event "Water Outlet Valve Open FVIR": Value Change {
        n35 = event-data() -> ()  [unwired: 1 in, 1 out]
        n36 = call-poly "Enqueue Message.vi"("error in (no error)"=w100, "Message"="WaterOutletOpenFVIR", "Message Queue"=w104) -> ("error out"=w102:errorcluster, "dup Message Queue"=w101:refnum<queue>)  [unwired: 7 in]
      }
      event "Water Outlet Valve Open LDO": Value Change {
        n37 = event-data() -> ()  [unwired: 1 in, 1 out]
        n38 = call-poly "Enqueue Message.vi"("error in (no error)"=w105, "Message"="WaterOutletOpenLDO", "Message Queue"=w109) -> ("error out"=w107:errorcluster, "dup Message Queue"=w106:refnum<queue>)  [unwired: 7 in]
      }
      event "Water Outlet Valve Close FVIR": Value Change {
        n39 = event-data() -> ()  [unwired: 1 in, 1 out]
        n40 = call-poly "Enqueue Message.vi"("error in (no error)"=w110, "Message"="WaterOutletCloseFVIR", "Message Queue"=w114) -> ("error out"=w112:errorcluster, "dup Message Queue"=w111:refnum<queue>)  [unwired: 7 in]
      }
      event "Water Outlet Valve Close LDO": Value Change {
        n41 = event-data() -> ()  [unwired: 1 in, 1 out]
        n42 = call-poly "Enqueue Message.vi"("error in (no error)"=w115, "Message"="WaterOutletCloseLDO", "Message Queue"=w119) -> ("error out"=w117:errorcluster, "dup Message Queue"=w116:refnum<queue>)  [unwired: 7 in]
      }
      event "Water Inlet Valve Open FVIR": Value Change {
        n43 = event-data() -> ()  [unwired: 1 in, 1 out]
        n44 = call-poly "Enqueue Message.vi"("error in (no error)"=w120, "Message"="WaterInletOpenFVIR", "Message Queue"=w124) -> ("error out"=w122:errorcluster, "dup Message Queue"=w121:refnum<queue>)  [unwired: 7 in]
      }
      event "Water Inlet Valve Open LDO": Value Change {
        n45 = event-data() -> ()  [unwired: 1 in, 1 out]
        n46 = call-poly "Enqueue Message.vi"("error in (no error)"=w125, "Message"="WaterInletOpenLDO", "Message Queue"=w129) -> ("error out"=w127:errorcluster, "dup Message Queue"=w126:refnum<queue>)  [unwired: 7 in]
      }
      event "Water Inlet Valve Close FVIR": Value Change {
        n47 = event-data() -> ()  [unwired: 1 in, 1 out]
        n48 = call-poly "Enqueue Message.vi"("error in (no error)"=w130, "Message"="WaterInletCloseFVIR", "Message Queue"=w134) -> ("error out"=w132:errorcluster, "dup Message Queue"=w131:refnum<queue>)  [unwired: 7 in]
      }
      event "Water Inlet Valve Close LDO": Value Change {
        n49 = event-data() -> ()  [unwired: 1 in, 1 out]
        n50 = call-poly "Enqueue Message.vi"("error in (no error)"=w135, "Message"="WaterInletCloseLDO", "Message Queue"=w139) -> ("error out"=w137:errorcluster, "dup Message Queue"=w136:refnum<queue>)  [unwired: 7 in]
      }
      event "Gas Solenoid Valve Open FVIR": Value Change {
        n51 = event-data() -> ()  [unwired: 1 in, 1 out]
        n52 = call-poly "Enqueue Message.vi"("error in (no error)"=w140, "Message"="GasSolenoidOpenFVIR", "Message Queue"=w144) -> ("error out"=w142:errorcluster, "dup Message Queue"=w141:refnum<queue>)  [unwired: 7 in]
      }
      event "Gas Solenoid Valve Open LDO": Value Change {
        n53 = event-data() -> ()  [unwired: 1 in, 1 out]
        n54 = call-poly "Enqueue Message.vi"("error in (no error)"=w145, "Message"="GasSolenoidOpenLDO", "Message Queue"=w149) -> ("error out"=w147:errorcluster, "dup Message Queue"=w146:refnum<queue>)  [unwired: 7 in]
      }
      event "Gas Solenoid Valve Close FVIR": Value Change {
        n55 = event-data() -> ()  [unwired: 1 in, 1 out]
        n56 = call-poly "Enqueue Message.vi"("error in (no error)"=w150, "Message"="GasSolenoidCloseFVIR", "Message Queue"=w154) -> ("error out"=w152:errorcluster, "dup Message Queue"=w151:refnum<queue>)  [unwired: 7 in]
      }
      event "Gas Solenoid Valve Close LDO": Value Change {
        n57 = event-data() -> ()  [unwired: 1 in, 1 out]
        n58 = call-poly "Enqueue Message.vi"("error in (no error)"=w155, "Message"="GasSolenoidCloseLDO", "Message Queue"=w159) -> ("error out"=w157:errorcluster, "dup Message Queue"=w156:refnum<queue>)  [unwired: 7 in]
      }
      event "Water Flow Intellifaucet DRK375 Open FVIR": Value Change {
        n59 = event-data() -> ()  [unwired: 1 in, 1 out]
        n60 = call-poly "Enqueue Message.vi"("error in (no error)"=w160, "Message"="WaterFlowOpenFVIR", "Message Queue"=w164) -> ("error out"=w162:errorcluster, "dup Message Queue"=w161:refnum<queue>)  [unwired: 7 in]
      }
      event "Water Flow Intellifaucet DRK375 Open LDO": Value Change {
        n61 = event-data() -> ()  [unwired: 1 in, 1 out]
        n62 = call-poly "Enqueue Message.vi"("error in (no error)"=w165, "Message"="WaterFlowStartLDO", "Message Queue"=w174) -> ("error out"=w167:errorcluster, "dup Message Queue"=w172:refnum<queue>)  [unwired: 7 in]
        n63 = for {
          N: 10 -> [_]
          tunnel: w167 -> [w175]
          tunnel: [w175] -> w166
          n64 = Wait Until Next ms Multiple(millisecond multiple=u32 100) -> ()  [unwired: 1 out]
        }
        n65 = call-poly "Enqueue Message.vi"("error in (no error)"=w166, "Message"="WaterFlowStartZeroLDO", "Message Queue"=w172) -> ("error out"=w170:errorcluster, "dup Message Queue"=w171:refnum<queue>)  [unwired: 7 in]
      }
      event "Water Flow Intellifaucet DRK375 Close FVIR": Value Change {
        n66 = event-data() -> ()  [unwired: 1 in, 1 out]
        n67 = call-poly "Enqueue Message.vi"("error in (no error)"=w177, "Message"="WaterFlowCloseFVIR", "Message Queue"=w181) -> ("error out"=w179:errorcluster, "dup Message Queue"=w178:refnum<queue>)  [unwired: 7 in]
      }
      event "Water Flow Intellifaucet DRK375 Close LDO": Value Change {
        n68 = event-data() -> ()  [unwired: 1 in, 1 out]
        n69 = call-poly "Enqueue Message.vi"("error in (no error)"=w182, "Message"="WaterFlowStopLDO", "Message Queue"=w191) -> ("error out"=w184:errorcluster, "dup Message Queue"=w188:refnum<queue>)  [unwired: 7 in]
        n70 = for {
          N: 10 -> [_]
          tunnel: w184 -> [w192]
          tunnel: [w192] -> w183
          n71 = Wait Until Next ms Multiple(millisecond multiple=u32 100) -> ()  [unwired: 1 out]
        }
        n72 = call-poly "Enqueue Message.vi"("error in (no error)"=w183, "Message"="WaterFlowStopZeroLDO", "Message Queue"=w188) -> ("error out"=w189:errorcluster, "dup Message Queue"=w187:refnum<queue>)  [unwired: 7 in]
      }
      event "Water Outlet Flow Proportional Valve EPV-312B Open FVIR": Value Change {
        n73 = event-data() -> ()  [unwired: 1 in, 1 out]
        n74 = call-poly "Enqueue Message.vi"("error in (no error)"=w194, "Message"="WaterFlowPropOpenFVIR", "Message Queue"=w198) -> ("error out"=w196:errorcluster, "dup Message Queue"=w195:refnum<queue>)  [unwired: 7 in]
      }
      event "Water Outlet Flow Proportional Valve EPV-312B Close FVIR": Value Change {
        n75 = event-data() -> ()  [unwired: 1 in, 1 out]
        n76 = call-poly "Enqueue Message.vi"("error in (no error)"=w199, "Message"="WaterFlowPropCloseFVIR", "Message Queue"=w203) -> ("error out"=w201:errorcluster, "dup Message Queue"=w200:refnum<queue>)  [unwired: 7 in]
      }
      event "Oil Spray 0.8 cc/min Open": Value Change {
        n77 = event-data() -> ()  [unwired: 1 in, 1 out]
        n78 = call-poly "Enqueue Message.vi"("error in (no error)"=w204, "Message"="OilSpray08Open", "Message Queue"=w208) -> ("error out"=w206:errorcluster, "dup Message Queue"=w205:refnum<queue>)  [unwired: 7 in]
      }
      event "Oil Spray 0.8 cc/min Close": Value Change {
        n79 = event-data() -> ()  [unwired: 1 in, 1 out]
        n80 = call-poly "Enqueue Message.vi"("error in (no error)"=w209, "Message"="OilSpray08Close", "Message Queue"=w213) -> ("error out"=w211:errorcluster, "dup Message Queue"=w210:refnum<queue>)  [unwired: 7 in]
      }
      event "Oil spray 0.8cc/min": Value Change {
        n81 = event-data() -> ("NewVal"=w219:bool)  [unwired: 1 in]
        n82 = case shown="False" w219 {
          tunnel: ["OilSpray08Close" ("Message") "OilSpray08Open" ("Message")] -> w215
          frame False {
          }
          frame True {
          }
        }
        n83 = call-poly "Enqueue Message.vi"("error in (no error)"=w214, "Message"=w215, "Message Queue"=w218) -> ("error out"=w217:errorcluster, "dup Message Queue"=w216:refnum<queue>)  [unwired: 7 in]
      }
      event "Oil Spray 1.1 cc/min Open": Value Change {
        n84 = event-data() -> ()  [unwired: 1 in, 1 out]
        n85 = call-poly "Enqueue Message.vi"("error in (no error)"=w222, "Message"="OilSpray11Open", "Message Queue"=w226) -> ("error out"=w224:errorcluster, "dup Message Queue"=w223:refnum<queue>)  [unwired: 7 in]
      }
      event "Oil Spray 1.1 cc/min Close": Value Change {
        n86 = event-data() -> ()  [unwired: 1 in, 1 out]
        n87 = call-poly "Enqueue Message.vi"("error in (no error)"=w227, "Message"="OilSpray11Close", "Message Queue"=w231) -> ("error out"=w229:errorcluster, "dup Message Queue"=w228:refnum<queue>)  [unwired: 7 in]
      }
      event "Oil spray 1.1cc/min": Value Change {
        n88 = event-data() -> ("NewVal"=w233:bool)  [unwired: 1 in]
        n89 = case shown="True" w233 {
          tunnel: ["OilSpray11Close" ("Message") "OilSpray11Open" ("Message")] -> w237
          frame False {
          }
          frame True {
          }
        }
        n90 = call-poly "Enqueue Message.vi"("error in (no error)"=w232, "Message"=w237, "Message Queue"=w236) -> ("error out"=w234:errorcluster, "dup Message Queue"=w235:refnum<queue>)  [unwired: 7 in]
      }
      event "Oil Spray 1.33 cc/min Open": Value Change {
        n91 = event-data() -> ()  [unwired: 1 in, 1 out]
        n92 = call-poly "Enqueue Message.vi"("error in (no error)"=w240, "Message"="OilSpray133Open", "Message Queue"=w244) -> ("error out"=w242:errorcluster, "dup Message Queue"=w241:refnum<queue>)  [unwired: 7 in]
      }
      event "Oil Spray 1.33 cc/min Close": Value Change {
        n93 = event-data() -> ()  [unwired: 1 in, 1 out]
        n94 = call-poly "Enqueue Message.vi"("error in (no error)"=w245, "Message"="OilSpray133Close", "Message Queue"=w249) -> ("error out"=w247:errorcluster, "dup Message Queue"=w246:refnum<queue>)  [unwired: 7 in]
      }
      event "Oil spray 1.33cc/min": Value Change {
        n95 = event-data() -> ("NewVal"=w251:bool)  [unwired: 1 in]
        n96 = case shown="True" w251 {
          tunnel: ["OilSpray133Close" ("Message") "OilSpray133Open" ("Message")] -> w255
          frame False {
          }
          frame True {
          }
        }
        n97 = call-poly "Enqueue Message.vi"("error in (no error)"=w250, "Message"=w255, "Message Queue"=w254) -> ("error out"=w252:errorcluster, "dup Message Queue"=w253:refnum<queue>)  [unwired: 7 in]
      }
      event "Heater ON": Value Change {
        n98 = event-data() -> ()  [unwired: 1 in, 1 out]
        n99 = call-poly "Enqueue Message.vi"("error in (no error)"=w258, "Message"="HeaterON", "Message Queue"=w262) -> ("error out"=w260:errorcluster, "dup Message Queue"=w259:refnum<queue>)  [unwired: 7 in]
      }
      event "Heater OFF": Value Change {
        n100 = event-data() -> ()  [unwired: 1 in, 1 out]
        n101 = call-poly "Enqueue Message.vi"("error in (no error)"=w263, "Message"="HeaterOFF", "Message Queue"=w267) -> ("error out"=w265:errorcluster, "dup Message Queue"=w264:refnum<queue>)  [unwired: 7 in]
      }
      event "Conveyor ON": Value Change {
        n102 = event-data() -> ()  [unwired: 1 in, 6 out]
        n103 = call-poly "Enqueue Message.vi"("error in (no error)"=w271, "Message"="ConveyorON", "Message Queue"=w269) -> ("error out"=w270:errorcluster, "dup Message Queue"=w268:refnum<queue>)  [unwired: 7 in]
      }
      event "Conveyor OFF": Value Change {
        n104 = event-data() -> ()  [unwired: 1 in, 6 out]
        n105 = call-poly "Enqueue Message.vi"("error in (no error)"=w276, "Message"="ConveyorOFF", "Message Queue"=w274) -> ("error out"=w275:errorcluster, "dup Message Queue"=w273:refnum<queue>)  [unwired: 7 in]
      }
      event "Blower ON": Value Change {
        n106 = event-data() -> ()  [unwired: 1 in, 6 out]
        n107 = call-poly "Enqueue Message.vi"("error in (no error)"=w281, "Message"="BlowerON", "Message Queue"=w279) -> ("error out"=w280:errorcluster, "dup Message Queue"=w278:refnum<queue>)  [unwired: 7 in]
      }
      event "Blower OFF": Value Change {
        n108 = event-data() -> ()  [unwired: 1 in, 6 out]
        n109 = call-poly "Enqueue Message.vi"("error in (no error)"=w286, "Message"="BlowerOFF", "Message Queue"=w284) -> ("error out"=w285:errorcluster, "dup Message Queue"=w283:refnum<queue>)  [unwired: 7 in]
      }
      event "Send parameters to PLC FVIR": Value Change {
        n110 = event-data() -> ()  [unwired: 1 in, 1 out]
        n111 = call-poly "Enqueue Message.vi"("error in (no error)"=w288, "Message"="SendParamToPLCFVIR", "Message Queue"=w292) -> ("error out"=w290:errorcluster, "dup Message Queue"=w289:refnum<queue>)  [unwired: 7 in]
      }
      event "Send parameters to PLC LDO": Value Change {
        n112 = event-data() -> ()  [unwired: 1 in, 1 out]
        n113 = call-poly "Enqueue Message.vi"("error in (no error)"=w293, "Message"="SendParamToPLCLDO", "Message Queue"=w297) -> ("error out"=w295:errorcluster, "dup Message Queue"=w294:refnum<queue>)  [unwired: 7 in]
      }
      event Panel Close? {
        # "Need to fix this!"
        # "Send the \"Exit\" message if the user closes the panel of the VI. Discard the event so the 'Confirm Quit' message has a chance to run."
        n114 = event-data() -> ()  [unwired: 1 in, 1 out]
        n115 = Stop(stop? (T)=TRUE) -> ()
        n116 = call-poly "Enqueue Message.vi"("Priority Message? (F)"=TRUE, "error in (no error)"=w299, "Message"="Exit", "Message Queue"=w303) -> ("error out"=w301:errorcluster, "dup Message Queue"=w302:refnum<queue>)  [unwired: 6 in]
        n117 = event-data("Discard?"=TRUE) -> ()  [unwired: 1 in, 1 out]
      }
      event Application Instance Close {
        n118 = event-data() -> ()  [unwired: 1 in, 1 out]
      }
      event User Event {
        w309 = "Exit" ("Exit String")
        # "The Message Handling Loop processed an \"Exit\" message, which fired this event to stop the Event Handling Loop."
        n119 = event-data() -> ()  [unwired: 1 in, 1 out]
        n120 = local write "General status for FVIR"(w309) -> ()
        n121 = local write "General status for LDO"(w309) -> ()
      }
      event Timeout {
        # "The timeout defines how frequencly data should be written to a logfile. When timeout is reach, a request for an additional Modbus read request is send to the Modbus Loop.\nThe shift register is used for checking if the \"Connect\" has been pressed or not."
        n122 = event-data() -> ()  [unwired: 1 in, 1 out]
        n123 = disable-structure shown="Enabled" {
          disable-tunnel: w317 -> [w323 w325]
          disable-tunnel: [w321 w324] -> w316
          disable-tunnel: [w320 w325] -> w314
          disable-tunnel: w313 -> [w319 w324]
          frame Disabled {
            n124 = call-poly "Enqueue Message.vi"("error in (no error)"=w323, "Message"="CheckBeforeWriteDataFVIR", "Message Queue"=w319) -> ("error out"=w320:errorcluster, "dup Message Queue"=w321:refnum<queue>)  [unwired: 7 in]
          }
          frame Enabled {
          }
        }
        n125 = call-poly "Enqueue Message.vi"("error in (no error)"=w314, "Message"="CheckBeforeWriteDataLDO", "Message Queue"=w316) -> ("error out"=w318:errorcluster, "dup Message Queue"=w312:refnum<queue>)  [unwired: 7 in]
      }
      event "Temp (°F)": Value Change {
        n126 = event-data() -> ()  [unwired: 1 in, 1 out]
        n127 = call-poly "Enqueue Message.vi"("Message Data"="Temp (°F)", "Message"="TempChangeDRK375", "Message Queue"=w328) -> ("error out"=w326:errorcluster)  [unwired: 7 in, 1 out]
      }
      event "Valve % Open": Value Change {
        n128 = event-data() -> ()  [unwired: 1 in, 1 out]
        n129 = call-poly "Enqueue Message.vi"("Message Data"="Valve % Open", "Message"="ValveChangeDRK375", "Message Queue"=w333) -> ("error out"=w331:errorcluster)  [unwired: 7 in, 1 out]
      }
      event "Proportioning Valve": Value Change {
        n130 = event-data() -> ()  [unwired: 1 in, 1 out]
        n131 = call-poly "Enqueue Message.vi"("Message Data"="Proportioning Valve", "Message"="ValveChangeEPV", "Message Queue"=w338) -> ("error out"=w336:errorcluster)  [unwired: 7 in, 1 out]
      }
      event "Gas Meter Tare Rate": Value Change {
        n132 = event-data() -> ()  [unwired: 1 in, 1 out]
        n133 = call-poly "Enqueue Message.vi"("Message"="Tare_Flow_LDO", "Message Queue"=w342) -> ("error out"=w341:errorcluster)  [unwired: 8 in, 1 out]
      }
      event "Gas Meter Tare Total": Value Change {
        n134 = event-data() -> ()  [unwired: 1 in, 1 out]
        n135 = call-poly "Enqueue Message.vi"("Message"="Tare_Totalizer_LDO", "Message Queue"=w346) -> ("error out"=w345:errorcluster)  [unwired: 8 in, 1 out]
      }
      event "Reset Flow Meter": Value Change {
        n136 = event-data() -> ()  [unwired: 1 in, 1 out]
        n137 = call "ResetFlowMeter.vi"("Queue in"=w350) -> ("error out 2"=w349:errorcluster)  [unwired: 10 in]
      }
      event "Burner": Value Change {
        n138 = event-data() -> ("NewVal"=w355:bool)  [unwired: 1 in, 5 out]
        n139 = case shown="False" w355 {
          tunnel: ["Water_Heater_Status_OFF_LDO" ("Message") "Water_Heater_Status_ON_LDO" ("Message")] -> w352
          frame False {
          }
          frame True {
          }
        }
        n140 = call-poly "Enqueue Message.vi"("Message"=w352, "Message Queue"=w353) -> ("error out"=w354:errorcluster)  [unwired: 8 in, 1 out]
      }
      event "Start recording data - LDO": Value Change {
        n141 = event-data() -> ("NewVal"=w360:bool)  [unwired: 1 in]
        n142 = case shown="True" w360 {
          tunnel: w362 -> [_ w366]
          tunnel: [w364 w365] -> w361
          tunnel: w359 -> [w364 _]
          frame False {
          }
          frame True {
            n143 = call-poly "Enqueue Message.vi"("Message"="Tare_Totalizer_LDO", "Message Queue"=w366) -> ("error out"=w365:errorcluster)  [unwired: 8 in, 1 out]
          }
        }
      }
    }
    n144 = call "Error Handler - Event Handling Loop.vi"("error in (no error)"=w44, "Message Queue"=w43) -> ("dup error in"=w45:errorcluster)  [unwired: 8 in, 1 out]
    "Event Loop" <- w39
  }
  n145 = while {
    tunnel: w20 -> [w391]
    tunnel: w27 -> [w395]
    shift-right: [w389] -> _
    shift-left: w32 -> [w390]
    tunnel: w3 -> [w394]
    tunnel: [w388] -> w37
    tunnel: w25 -> [w385]
    tunnel: w26 -> [w384]
    tunnel: w2 -> [w383]
    shift-right: [w382] -> _
    shift-left: _ -> [w381]
    tunnel: w18 -> [w380]
    tunnel: w15 -> [w379]
    shift-right: [w378] -> _
    shift-left: w16 -> [w377]
    tunnel: w14 -> [w376]
    tunnel: w6 -> [w375]
    shift-right: [w372] -> _
    shift-left: T1 {"Burner ON"=FALSE, "0.8 ml Bool"=FALSE, "1.1 Bool"=FALSE, "1.33 Bool"=FALSE, "Start recording data-LDO"=FALSE} -> [w373]
    shift-right: [w369] -> _
    shift-left: string[] [] -> [w371]
    i -> [w374]
    stop <- w396 stop-if-true
    # "UI Message Loop"
    n146 = call "Dequeue Message.vi"("error in (no error)"=w394, "Message Queue"=w391) -> ("error out"=w393:errorcluster, "Message Data"=w392:variant, "Message"=w370:string, "dup Message Queue"=w386:refnum<queue>)  [unwired: 6 in]
    n147 = case "Message Cases" shown="\"DisplayValuesFromPLC\"" w370 {
      selector: w370 -> [_ _ _ _ _ _ _ _ _ _ _ _ _ _ _ _ _ _ _ _ _ _ _ _ _ _ _ _ _ _ _ _ _ _ _ _ _ _ _ _ _ _ _ _ _ _ _ _ _ _ _ _ _ _ _ _ _ _ _ _ _ _ _ _ _ _ w1505]
      tunnel: w386 -> [w416 _ _ _ _ w516 w534 _ w573 w597 w689 w700 w712 w724 w732 w752 w772 w792 w816 w828 w840 w852 w864 w876 w888 w900 w912 w924 w936 w948 w960 w972 w984 w996 w1008 w1020 w1032 w1044 w1051 w1063 w1080 w1092 w1104 w1116 w1128 w1140 w1152 w1164 w1171 w1182 w1196 w1208 w1230 w1260 w1270 w1300 _ w1397 w1408 w1418 w1432 _ _ _ _ _ _]
      tunnel: w393 -> [w415 w425 w482 w492 w502 w515 w531 w548 w559 w593 w683 w702 w714 w726 w735 w755 w775 w795 w817 w829 w841 w853 w865 w877 w889 w901 w913 w925 w937 w949 w961 w973 w985 w997 w1009 w1021 w1033 w1045 w1054 w1066 w1081 w1093 w1105 w1117 w1129 w1141 w1153 w1165 w1174 w1186 w1198 w1210 w1231 w1261 w1278 w1322 w1365 w1400 w1411 w1424 w1437 w1445 w1454 w1461 w1481 w1500 _]
      tunnel: [w409 w425 w483 w493 w503 w511 w537 w548 w568 w590 w688 w697 w709 w720 w738 w758 w778 w798 w819 w831 w843 w855 w867 w879 w891 w903 w915 w927 w939 w951 w963 w975 w987 w999 w1011 w1023 w1035 w1047 w1053 w1065 w1083 w1095 w1107 w1119 w1131 w1143 w1155 w1167 w1173 w1185 w1197 w1209 w1233 w1239 w1279 w1301 w1364 w1382 w1406 w1419 w1433 w1444 w1453 w1463 w1492 w1499 w1504] -> w387
      tunnel: [_ _ _ _ _ _ _ _ _ _ _ _ _ _ _ _ _ _ _ _ _ _ _ _ _ _ _ _ _ _ _ _ _ _ _ _ _ _ _ _ _ _ _ _ _ _ _ _ _ _ _ _ _ _ _ _ _ _ _ _ _ _ _ _ TRUE _ _] -> w396
      tunnel: w392 -> [_ _ w481 w491 w501 _ _ _ _ _ _ _ _ _ _ _ _ _ _ _ _ _ _ _ _ _ _ _ _ _ _ _ _ _ _ _ _ _ _ _ _ _ _ _ _ _ _ _ _ _ _ _ _ _ w1277 _ _ w1399 w1410 w1422 w1436 _ _ w1464 w1489 _ _]
      tunnel: w395 -> [_ _ _ _ _ _ _ _ _ _ _ _ _ _ _ _ _ _ _ _ _ _ _ _ _ _ _ _ _ _ _ _ _ _ _ _ _ _ _ _ _ _ _ _ _ _ _ _ _ _ _ _ _ _ _ _ _ _ _ _ _ _ _ _ w1493 _ _]
      tunnel: w390 -> [w420 w427 w477 w487 w499 w512 w527 w550 w570 w599 w692 w704 w716 w728 w733 w753 w773 w793 w814 w826 w838 w850 w862 w874 w886 w898 w910 w922 w934 w946 w958 w970 w982 w994 w1006 w1018 w1030 w1042 w1060 w1072 w1079 w1091 w1103 w1115 w1127 w1139 w1150 w1162 w1180 w1192 w1204 w1216 w1228 w1259 w1275 w1352 w1368 w1390 w1413 w1426 w1439 w1448 w1457 w1467 w1491 w1498 w1506]
      tunnel: [w420 w426 w477 w487 w499 w512 w527 w550 w570 w599 w692 w704 w716 w728 w733 w753 w773 w793 w814 w826 w838 w850 w862 w874 w886 w898 w910 w922 w934 w946 w958 w970 w982 w994 w1006 w1018 w1030 w1042 w1060 w1072 w1079 w1091 w1103 w1115 w1127 w1139 w1150 w1162 w1180 w1192 w1204 w1216 w1228 w1259 w1275 w1352 w1368 w1390 w1413 w1426 w1439 w1448 w1457 w1467 w1491 w1498 w1506] -> w389
      tunnel: w385 -> [w404 _ _ _ _ _ _ _ w572 w596 w674 w703 w715 w727 w734 w754 w774 w794 w815 w827 w839 w851 w863 w875 w887 w899 w911 w923 w935 w947 w959 w971 w983 w995 w1007 w1019 w1031 w1043 w1052 w1064 _ _ _ _ _ _ w1151 w1163 w1172 w1181 w1195 w1207 w1229 w1238 _ _ w1366 _ _ _ _ _ _ _ w1487 _ _]
      tunnel: w384 -> [_ _ _ _ _ w509 w529 _ w571 _ _ _ _ _ _ _ _ _ _ _ _ _ _ _ _ _ _ _ _ _ _ _ _ _ _ _ _ _ _ _ _ _ _ _ _ _ _ _ _ _ _ _ _ _ _ _ _ _ _ _ _ _ _ _ w1485 _ _]
      tunnel: w383 -> [_ _ _ _ _ _ _ _ w566 w589 w687 _ _ _ _ _ _ _ _ _ _ _ _ _ _ _ _ _ _ _ _ _ _ _ _ _ _ _ _ _ _ _ _ _ _ _ _ _ _ _ _ _ _ _ _ _ _ _ _ _ _ w1443 w1452 _ w1483 _ _]
      tunnel: [FALSE w424 w476 w486 w496 w506 w528 FALSE w553 FALSE w684 w695 w707 w719 w731 w751 w771 w791 w811 w823 w835 w847 w859 w871 w883 w895 w907 w919 w931 w943 w955 w967 w979 w991 w1003 w1015 w1027 w1039 w1059 w1071 w1076 w1088 w1100 w1112 w1124 w1136 w1147 w1159 w1179 w1191 w1203 w1215 w1219 w1244 w1267 w1351 w1367 w1395 w1412 w1425 w1438 w1447 w1456 w1460 w1482 w1497 w1503] -> w382
      tunnel: w381 -> [_ w424 w476 w486 w496 w506 w528 _ w553 _ w684 w695 w707 w719 w731 w751 w771 w791 w811 w823 w835 w847 w859 w871 w883 w895 w907 w919 w931 w943 w955 w967 w979 w991 w1003 w1015 w1027 w1039 w1059 w1071 w1076 w1088 w1100 w1112 w1124 w1136 w1147 w1159 w1179 w1191 w1203 w1215 w1219 w1244 w1269 w1351 w1367 w1395 w1412 w1425 w1438 w1447 w1456 w1460 w1482 w1497 w1503]
      tunnel: w380 -> [_ _ _ _ _ _ _ _ _ _ _ _ _ _ _ _ _ _ _ _ _ _ _ _ _ _ _ _ _ _ _ _ _ _ _ _ _ _ _ _ w1075 w1087 w1099 w1111 w1123 w1135 _ _ _ _ _ _ _ _ _ _ _ _ _ _ _ _ _ _ w1479 _ _]
      tunnel: w379 -> [w403 _ _ _ _ _ _ _ _ _ w672 _ _ _ _ _ _ _ _ _ _ _ _ _ _ _ _ _ _ _ _ _ _ _ _ _ _ _ _ _ _ _ _ _ _ _ _ _ _ _ _ _ _ _ _ _ _ _ _ _ _ _ _ _ w1477 _ _]
      tunnel: w377 -> [w411 w423 w475 w485 w495 w505 w526 w547 w552 w585 w680 w694 w706 w718 w730 w750 w770 w790 w810 w822 w834 w846 w858 w870 w882 w894 w906 w918 w930 w942 w954 w966 w978 w990 w1002 w1014 w1026 w1038 w1050 w1062 w1074 w1086 w1098 w1110 w1122 w1134 w1146 w1158 w1169 w1184 w1194 w1205 w1218 w1243 w1266 w1314 w1358 w1380 w1404 w1417 w1431 w1441 w1450 w1459 w1476 w1496 w1502]
      tunnel: [w411 w423 w475 w485 w495 w505 w526 w547 w552 w585 w680 w694 w706 w718 w730 w750 w770 w790 w810 w822 w834 w846 w858 w870 w882 w894 w906 w918 w930 w942 w954 w966 w978 w990 w1002 w1014 w1026 w1038 w1050 w1062 w1074 w1086 w1098 w1110 w1122 w1134 w1146 w1158 w1169 w1184 w1194 w1205 w1218 w1243 w1266 w1318 w1358 w1378 w1403 w1416 w1430 w1441 w1450 w1459 w1476 w1496 w1502] -> w378
      tunnel: w376 -> [_ _ _ _ _ _ _ _ _ _ _ _ _ _ _ _ _ _ _ _ _ _ _ _ _ _ _ _ _ _ _ _ _ _ _ _ _ _ _ _ _ _ _ _ _ _ _ _ _ _ _ _ _ _ _ _ _ _ _ _ _ _ _ _ w1474 _ _]
      tunnel: w375 -> [_ _ _ _ _ _ _ _ _ _ _ _ _ _ _ _ _ _ _ _ _ _ _ _ _ _ _ _ _ _ _ _ _ _ _ _ _ _ _ _ _ _ _ _ _ _ _ _ _ _ _ _ _ _ _ _ _ _ _ _ _ _ _ _ w1470 _ _]
      tunnel: w373 -> [w410 w422 w474 w484 w494 w504 w525 w546 w551 w586 w681 w693 w705 w717 w729 w749 w769 w789 w809 w821 w833 w845 w857 w869 w881 w893 w905 w917 w929 w941 w953 w965 w977 w989 w1001 w1013 w1025 w1037 w1049 w1061 w1073 w1085 w1097 w1109 w1121 w1133 w1145 w1157 w1170 w1183 w1193 w1206 w1217 w1242 w1265 w1309 w1359 w1377 w1401 w1414 w1427 w1442 w1451 w1458 w1468 w1495 w1501]
      tunnel: [w410 w422 w474 w484 w494 w504 w525 w546 w551 w586 w681 w693 w705 w717 w729 w749 w769 w789 w809 w821 w833 w845 w857 w869 w881 w893 w905 w917 w929 w941 w953 w965 w977 w989 w1001 w1013 w1025 w1037 w1049 w1061 w1073 w1085 w1097 w1109 w1121 w1133 w1145 w1157 w1170 w1183 w1193 w1206 w1217 w1242 w1265 w1296 w1359 w1377 w1401 w1414 w1427 w1442 w1451 w1458 w1468 w1495 w1501] -> w372
      frame "Initialize" {
        # "Using this flag for checking if the value of the logfile of % Butane is above 1.8. If this is true, this flag will be set to TRUE, if not, it is set to FALSE. This is usefull in the \"StopTestFVIR\" when the value is above 1.8. Because otherwise this will be equal to that the \"STOP\" button will be pressed all the time, and we just want it to be pressed ones."
        # "Reset all values of the HMI"
        # "Initialize - Get configuration settings, then message the UI to initialize, and broadcast the settings to the other message loops."
        n148 = call-poly "Enqueue Message.vi"("error in (no error)"=w415, "Message Data"=u16[] [0, 0, 0, 0, 0, 0, 0, 0] ("Input Registers"), "Message"="DisplayValuesFromPLC", "Message Queue"=w416) -> ("error out"=w414:errorcluster, "dup Message Queue"=w413:refnum<queue>)  [unwired: 6 in]
        n149 = call-poly "Enqueue Message.vi"("error in (no error)"=w414, "Message"="Init UI Refs", "Message Queue"=w413) -> ("error out"=w405:errorcluster, "dup Message Queue"=w406:refnum<queue>)  [unwired: 7 in]
        n150 = call "FVIR_Setup_Parameters.vi"("error in (no error)"=w405, "UI in"=w406) -> ("error out"=w407:errorcluster, "UI out"=w408:refnum<queue>)  [unwired: 8 in]
        n151 = call "LDO_Setup_Parameters.vi"("Temp (°F) - Automatic Mode"="Temp (°F) - Automatic Mode", "Alicat_GasMeter"=w403, "Valve % Open - Automatic Mode"="Valve % Open - Automatic Mode", "Modbus"=w404, "error in (no error)"=w407, "UI in"=w408) -> ("error out"=w409:errorcluster)  [unwired: 5 in]
      }
      frame "Init UI Refs" {
        # "Init UI Refs - Store control references for UI controls.  Also enable/disable controls appropriately."
        n152 = disable-structure shown="Enabled" {
          disable-tunnel: w427 -> [w472 w473]
          disable-tunnel: [w471 w473] -> w426
          frame Disabled {
            n153 = control-ref of="Start"() -> (w468:refnum<vi>)
            n154 = control-ref of="Stop"() -> (w450:refnum<vi>)
            n155 = control-ref of="Start Test Case FVIR"() -> (w451:refnum<vi>)
            n156 = control-ref of="Stop Test Case FVIR"() -> (w465:refnum<vi>)
            n157 = control-ref of="Water Outlet Valve Open FVIR"() -> (w464:refnum<vi>)
            n158 = control-ref of="Water Outlet Valve Close FVIR"() -> (w463:refnum<vi>)
            n159 = control-ref of="Water Inlet Valve Open FVIR"() -> (w462:refnum<vi>)
            n160 = control-ref of="Water Inlet Valve Close FVIR"() -> (w461:refnum<vi>)
            n161 = control-ref of="Gas Solenoid Valve Open FVIR"() -> (w452:refnum<vi>)
            n162 = control-ref of="Gas Solenoid Valve Close FVIR"() -> (w453:refnum<vi>)
            n163 = control-ref of="Water Flow Intellifaucet DRK375 Open FVIR"() -> (w454:refnum<vi>)
            n164 = control-ref of="Water Flow Intellifaucet DRK375 Close FVIR"() -> (w455:refnum<vi>)
            n165 = control-ref of="Spill can - Go to Home Pos"() -> (w456:refnum<vi>)
            n166 = control-ref of="Spill can - Go to Work Pos"() -> (w457:refnum<vi>)
            n167 = control-ref of="Move mannequin - Go to Home Pos"() -> (w458:refnum<vi>)
            n168 = control-ref of="Move mannequin - Go to Work Pos"() -> (w459:refnum<vi>)
            n169 = control-ref of="Send parameters to PLC FVIR"() -> (w449:refnum<vi>)
            n170 = control-ref of="Water Outlet Flow Proportional Valve EPV-312B Open FVIR"() -> (w448:refnum<vi>)
            n171 = control-ref of="Water Outlet Flow Proportional Valve EPV-312B Close FVIR"() -> (w447:refnum<vi>)
            n172 = control-ref of="Start Test Case LDO"() -> (w446:refnum<vi>)
            n173 = control-ref of="Stop Test Case LDO"() -> (w445:refnum<vi>)
            n174 = control-ref of="Water Outlet Valve Open LDO"() -> (w444:refnum<vi>)
            n175 = control-ref of="Water Outlet Valve Close LDO"() -> (w443:refnum<vi>)
            n176 = control-ref of="Water Inlet Valve Open LDO"() -> (w442:refnum<vi>)
            n177 = control-ref of="Water Inlet Valve Close LDO"() -> (w441:refnum<vi>)
            n178 = control-ref of="Gas Solenoid Valve Open LDO"() -> (w440:refnum<vi>)
            n179 = control-ref of="Gas Solenoid Valve Close LDO"() -> (w439:refnum<vi>)
            n180 = control-ref of="Water Flow Intellifaucet DRK375 Open LDO"() -> (w438:refnum<vi>)
            n181 = control-ref of="Water Flow Intellifaucet DRK375 Close LDO"() -> (w437:refnum<vi>)
            n182 = control-ref of="Oil Spray 0.8 cc/min Open"() -> (w436:refnum<vi>)
            n183 = control-ref of="Oil Spray 0.8 cc/min Close"() -> (w435:refnum<vi>)
            n184 = control-ref of="Oil Spray 1.1 cc/min Open"() -> (w434:refnum<vi>)
            n185 = control-ref of="Oil Spray 1.1 cc/min Close"() -> (w433:refnum<vi>)
            n186 = control-ref of="Oil Spray 1.33 cc/min Open"() -> (w432:refnum<vi>)
            n187 = control-ref of="Oil Spray 1.33 cc/min Close"() -> (w431:refnum<vi>)
            n188 = control-ref of="Heater ON"() -> (w430:refnum<vi>)
            n189 = control-ref of="Heater OFF"() -> (w429:refnum<vi>)
            n190 = control-ref of="Select test case"() -> (w460:refnum<vi>)
            n191 = control-ref of="General status for FVIR"() -> (w428:refnum<vi>)
            n192 = Build Array(w429, w430, w431, w432, w433, w434, w435, w436, w437, w438, w439, w440, w441, w442, w443, w444, w445, w446, w447, w448, w449, w460, w459, w458, w457, w456, w455, w454, w453, w452, w461, w462, w463, w464, w465, w451, w450) -> (w467:refnum<vi>[])
            n193 = Build Array(w468) -> (w466:refnum<vi>[])
            n194 = call "Set Enable State on Multiple Controls.vi"("Enable?"=FALSE, "Controls"=w467) -> ()  [unwired: 10 in]
            n195 = call "Set Enable State on Multiple Controls.vi"("Enable?"=TRUE, "Controls"=w466) -> ()  [unwired: 10 in]
            n196 = Bundle By Name(cluster=w472, "Start Ref"=w468, "Stop Ref"=w450, "Status Ref"=w428, "Start test case FVIR Ref"=w451, "Stop test case FVIR Ref"=w465, "Water Outlet Valve Open FVIR Ref"=w464, "Water Outlet Valve Close FVIR Ref"=w463, "Water Inlet Valve Open FVIR Ref"=w462, "Water Inlet Valve Close FVIR Ref"=w461, "Gas Solenoid Valve Open FVIR Ref"=w452, "Gas Solenoid Valve Close FVIR Ref"=w453, "Water Flow Open FVIR Ref"=w454, "Water Flow Close FVIR Ref"=w455, "Spill can Home pos Ref"=w456, "Spill can Work pos Ref"=w457, "Move Mannequin Home pos Ref"=w458, "Move Mannequin Work pos Ref"=w459, "Listbox Ref"=w460, "Send Param to PLC FVIR Ref"=w449, "Water Flow Prop Open FVIR Ref"=w448, "Water Flow Prop Close FVIR Ref"=w447, "Start test case LDO Ref"=w446, "Stop test case LDO Ref"=w445, "Water Outlet Valve Open LDO Ref"=w444, "Water Outlet Valve Close LDO Ref"=w443, "Water Inlet Valve Open LDO Ref"=w442, "Water Inlet Valve Close LDO Ref"=w441, "Gas Solenoid Valve Open LDO Ref"=w440, "Gas Solenoid Valve Close LDO Ref"=w439, "Water Flow Open LDO Ref"=w438, "Water Flow Close LDO Ref"=w437, "Oil spray 0.8cc/min Open Ref"=w436, "Oil spray 0.8cc/min Close Ref"=w435, "Oil spray 1.1cc/min Open Ref"=w434, "Oil spray 1.1cc/min Close Ref"=w433, "Oil spray 1.33cc/min Open Ref"=w432, "Oil spray 1.33cc/min Close Ref"=w431, "Heater ON Ref"=w430, "Heater OFF Ref"=w429) -> (w471:T11)
          }
          frame Enabled {
          }
        }
        n197 = property on="Stop Test Case LDO" class="Bool"("DisabledEnum"=T13."Enabled" ("Disabled")) -> ()  [unwired: 2 in, 2 out]
      }
      frame "Update status - FVIR" {
        # "Update Status - Convert the message data to a string to display in the Status indicator."
        n198 = Variant To Data(error in=w482, type="", Variant=w481) -> (data=→"General status for FVIR":string, error out=w479:errorcluster)
        n199 = Merge Errors(w479) -> (w483:errorcluster)
      }
      frame "Update status - LDO" {
        # "Update Status - Convert the message data to a string to display in the Status indicator."
        n200 = Variant To Data(error in=w492, type="", Variant=w491) -> (data=→"General status for LDO":string, error out=w489:errorcluster)
        n201 = Merge Errors(w489) -> (w493:errorcluster)
      }
      frame "ShowLabViewLifeBit" {
        # "Update Status - Convert the message data to a string to display in the Status indicator."
        n202 = Variant To Data(error in=w502, type=TRUE, Variant=w501) -> (data=→"Labview lifebit":bool, error out=w500:errorcluster)
        n203 = Merge Errors(w500) -> (w503:errorcluster)
      }
      frame "Start" {
        # "Note: So right now, I am writing to the HMI that we only read the log file. \nHowever the acqusition and logging from the original template does also happens, which needs to be \ncleaned up later."
        # "Start - Enable/Disable buttons appropriately for an acquisition that has started, and update status display."
        n204 = disable-structure shown="Disabled" {
          disable-tunnel: w512 -> [w524 _]
          frame Disabled {
            # "Enable: Stop\nDisable: Start, Exit, Settings"
            n205 = Unbundle By Name(w524) -> ("Stop Ref"=w519:refnum<vi>, "Start Ref"=w518:refnum<vi>, "Exit Ref"=w517:refnum<vi>)
            n206 = Build Array(w518, w517) -> (w522:refnum<vi>[])
            n207 = Build Array(w519) -> (w521:refnum<vi>[])
            n208 = call "Set Enable State on Multiple Controls.vi"("Enable?"=FALSE, "Controls"=w522) -> ()  [unwired: 10 in]
            n209 = call "Set Enable State on Multiple Controls.vi"("Enable?"=TRUE, "Controls"=w521) -> ()  [unwired: 10 in]
          }
          frame Enabled {
          }
        }
        n210 = call-poly "Enqueue Message.vi"("error in (no error)"=w515, "Message Data"="Starting to read log file..." ("Acquiring and Logging..."), "Message"="Update Status - FVIR", "Message Queue"=w516) -> ("error out"=w508:errorcluster)  [unwired: 6 in, 1 out]
        n211 = call-poly "Enqueue Message.vi"("error in (no error)"=w508, "Message Data"="Path to local logfile", "Message"="Start", "Message Queue"=w509) -> ("error out"=w511:errorcluster)  [unwired: 6 in, 1 out]
      }
      frame "Stop" {
        # "Stop - Enable/Disable buttons appropriately for an acquisition that has stopped, and update status display."
        n212 = disable-structure shown="Disabled" {
          disable-tunnel: w527 -> [w538 _]
          frame Disabled {
            n213 = Unbundle By Name(w538) -> ("Stop Ref"=w544:refnum<vi>, "Start Ref"=w542:refnum<vi>, "Exit Ref"=w541:refnum<vi>)
            n214 = Build Array(w544) -> (w540:refnum<vi>[])
            n215 = Build Array(w542, w541) -> (w539:refnum<vi>[])
            n216 = call "Set Enable State on Multiple Controls.vi"("Enable?"=FALSE, "Controls"=w540) -> ()  [unwired: 10 in]
            n217 = call "Set Enable State on Multiple Controls.vi"("Enable?"=TRUE, "Controls"=w539) -> ()  [unwired: 10 in]
          }
          frame Enabled {
          }
        }
        n218 = call-poly "Enqueue Message.vi"("error in (no error)"=w531, "Message Data"="Stopping to read log file..." ("Acquiring and Logging..."), "Message"="Update Status - FVIR", "Message Queue"=w534) -> ("error out"=w530:errorcluster)  [unwired: 6 in, 1 out]
        n219 = call-poly "Enqueue Message.vi"("error in (no error)"=w530, "Message"="Stop", "Message Queue"=w529) -> ("error out"=w536:errorcluster)  [unwired: 7 in, 1 out]
        n220 = Merge Errors(w536) -> (w537:errorcluster)
      }
      frame "Connect" {
        # "Start - Enable/Disable buttons appropriately for an acquisition that has started, and update status display."
      }
      frame "Disconnect" {
        w567 = "Disconnect" ("Message")
        # "Sending an \"init\" so \nthat all the buttons gets back to disabled"
        # "Enable: Connect\nDisable: Disconnect, Move mannequin, Spill Can, Water Outlet Valve, Exit"
        # "Message Modbus Message and RedDataFile loops to disconnect."
        # "Start - Enable/Disable buttons appropriately for an acquisition that has started, and update status display."
        n221 = disable-structure shown="Disabled" {
          disable-tunnel: w570 -> [w579 _]
          frame Disabled {
            n222 = Unbundle By Name(w579) -> ("Disconnect Ref"=w578:refnum<vi>, "Connect Ref"=w576:refnum<vi>, "Exit Ref"=w575:refnum<vi>)
            n223 = Build Array(w578) -> (w581:refnum<vi>[])
            n224 = Build Array(w576, w575) -> (w574:refnum<vi>[])
            n225 = call "Set Enable State on Multiple Controls.vi"("Enable?"=FALSE, "Controls"=w581) -> ()  [unwired: 10 in]
            n226 = call "Set Enable State on Multiple Controls.vi"("Enable?"=TRUE, "Controls"=w574) -> ()  [unwired: 10 in]
          }
          frame Enabled {
          }
        }
        n227 = call-poly "Enqueue Message.vi"("error in (no error)"=w559, "Message Data"="Disconnecting with Modbus TCP/IP..." ("Acquiring and Logging..."), "Message"="Update Status - FVIR", "Message Queue"=w573) -> ("error out"=w558:errorcluster, "dup Message Queue"=w563:refnum<queue>)  [unwired: 6 in]
        n228 = call-poly "Enqueue Message.vi"("error in (no error)"=w558, "Message Data"="Disconnecting with Modbus TCP/IP..." ("Acquiring and Logging..."), "Message"="Update Status - LDO", "Message Queue"=w563) -> ("error out"=w562:errorcluster, "dup Message Queue"=w561:refnum<queue>)  [unwired: 6 in]
        n229 = call-poly "Enqueue Message.vi"("error in (no error)"=w562, "Message"="Init UI Refs", "Message Queue"=w561) -> ("error out"=w557:errorcluster)  [unwired: 7 in, 1 out]
        n230 = call-poly "Enqueue Message.vi"("error in (no error)"=w557, "Message"=w567, "Message Queue"=w572) -> ("error out"=w556:errorcluster)  [unwired: 7 in, 1 out]
        n231 = call-poly "Enqueue Message.vi"("error in (no error)"=w556, "Message"=w567, "Message Queue"=w571) -> ("error out"=w555:errorcluster)  [unwired: 7 in, 1 out]
        n232 = call-poly "Enqueue Message.vi"("error in (no error)"=w555, "Message"=w567, "Message Queue"=w566) -> ("error out"=w568:errorcluster)  [unwired: 7 in, 1 out]
      }
      frame "StartTestCaseFVIR" {
        # "When the operator starts a test, the information about \nthe test is passed to the Writing DataFile Loop"
        # "Indicate that now a FVIR test is active"
        # "Start - Enable/Disable buttons appropriately for an acquisition that has started, and update status display."
        n233 = call-poly "Enqueue Message.vi"("error in (no error)"=w593, "Message"="StartTestFVIR", "Message Queue"=w596) -> ("error out"=w592:errorcluster, "dup Message Queue"=w595:refnum<queue>)  [unwired: 7 in]
        n234 = case shown="0, Default" "Select test case" {
          tunnel: w597 -> [w606 w615 w624 w633 w642 w651 w660 w669]
          tunnel: w592 -> [w605 w614 w623 w632 w641 w650 w659 w668]
          tunnel: w595 -> [w603 w612 w621 w630 w639 w648 w657 w666]
          tunnel: [w602 w611 w620 w629 w638 w647 w656 w665] -> w591
          tunnel: ["FV_case_1_Winter" ("Acquiring and Logging...") "FV_ case _1_Summer" ("Acquiring and Logging...") "FV_case _2_Winter" ("Acquiring and Logging...") "FV_case_2_Summer" ("Acquiring and Logging...") "FV_case_3_Winter" ("Acquiring and Logging...") "FV_case_3_Summer" ("Acquiring and Logging...") "FV_case_4_Winter" ("Acquiring and Logging...") "FV_case _4_Summer" ("Acquiring and Logging...")] -> w584
          frame 0, Default {
            n235 = call-poly "Enqueue Message.vi"("error in (no error)"=w605, "Message Data"="Test case #1 - Winter has started ..." ("Acquiring and Logging..."), "Message"="Update Status - FVIR", "Message Queue"=w606) -> ("error out"=w604:errorcluster)  [unwired: 6 in, 1 out]
            n236 = call-poly "Enqueue Message.vi"("error in (no error)"=w604, "Message"="TestCase1Winter", "Message Queue"=w603) -> ("error out"=w602:errorcluster)  [unwired: 7 in, 1 out]
          }
          frame 1 {
            n237 = call-poly "Enqueue Message.vi"("error in (no error)"=w614, "Message Data"="Test case #1 - Summer has started ..." ("Acquiring and Logging..."), "Message"="Update Status - FVIR", "Message Queue"=w615) -> ("error out"=w613:errorcluster)  [unwired: 6 in, 1 out]
            n238 = call-poly "Enqueue Message.vi"("error in (no error)"=w613, "Message"="TestCase1Summer", "Message Queue"=w612) -> ("error out"=w611:errorcluster)  [unwired: 7 in, 1 out]
          }
          frame 2 {
            n239 = call-poly "Enqueue Message.vi"("error in (no error)"=w623, "Message Data"="Test case #2 - Winter has started ..." ("Acquiring and Logging..."), "Message"="Update Status - FVIR", "Message Queue"=w624) -> ("error out"=w622:errorcluster)  [unwired: 6 in, 1 out]
            n240 = call-poly "Enqueue Message.vi"("error in (no error)"=w622, "Message"="TestCase2Winter", "Message Queue"=w621) -> ("error out"=w620:errorcluster)  [unwired: 7 in, 1 out]
          }
          frame 3 {
            n241 = call-poly "Enqueue Message.vi"("error in (no error)"=w632, "Message Data"="Test case #2 - Summer has started ..." ("Acquiring and Logging..."), "Message"="Update Status - FVIR", "Message Queue"=w633) -> ("error out"=w631:errorcluster)  [unwired: 6 in, 1 out]
            n242 = call-poly "Enqueue Message.vi"("error in (no error)"=w631, "Message"="TestCase2Summer", "Message Queue"=w630) -> ("error out"=w629:errorcluster)  [unwired: 7 in, 1 out]
          }
          frame 4 {
            n243 = call-poly "Enqueue Message.vi"("error in (no error)"=w641, "Message Data"="Test case #3 - Winter has started ..." ("Acquiring and Logging..."), "Message"="Update Status - FVIR", "Message Queue"=w642) -> ("error out"=w640:errorcluster)  [unwired: 6 in, 1 out]
            n244 = call-poly "Enqueue Message.vi"("error in (no error)"=w640, "Message"="TestCase3Winter", "Message Queue"=w639) -> ("error out"=w638:errorcluster)  [unwired: 7 in, 1 out]
          }
          frame 5 {
            n245 = call-poly "Enqueue Message.vi"("error in (no error)"=w650, "Message Data"="Test case #3 - Summer has started ..." ("Acquiring and Logging..."), "Message"="Update Status - FVIR", "Message Queue"=w651) -> ("error out"=w649:errorcluster)  [unwired: 6 in, 1 out]
            n246 = call-poly "Enqueue Message.vi"("error in (no error)"=w649, "Message"="TestCase3Summer", "Message Queue"=w648) -> ("error out"=w647:errorcluster)  [unwired: 7 in, 1 out]
          }
          frame 6 {
            n247 = call-poly "Enqueue Message.vi"("error in (no error)"=w659, "Message Data"="Test case #4 - Winter has started ..." ("Acquiring and Logging..."), "Message"="Update Status - FVIR", "Message Queue"=w660) -> ("error out"=w658:errorcluster)  [unwired: 6 in, 1 out]
            n248 = call-poly "Enqueue Message.vi"("error in (no error)"=w658, "Message"="TestCase4Winter", "Message Queue"=w657) -> ("error out"=w656:errorcluster)  [unwired: 7 in, 1 out]
          }
          frame 7 {
            n249 = call-poly "Enqueue Message.vi"("error in (no error)"=w668, "Message Data"="Test case #4 - Summer has started ..." ("Acquiring and Logging..."), "Message"="Update Status - FVIR", "Message Queue"=w669) -> ("error out"=w667:errorcluster)  [unwired: 6 in, 1 out]
            n250 = call-poly "Enqueue Message.vi"("error in (no error)"=w667, "Message"="TestCase4Summer", "Message Queue"=w666) -> ("error out"=w665:errorcluster)  [unwired: 7 in, 1 out]
          }
        }
        n251 = Bundle By Name(cluster=w585, "PLC Data Out.Data to Save.Test Case - FVIR"=w584) -> (w583:T2)
        n252 = Unbundle By Name(w583) -> ("PLC Data Out"=w582:T3)
        n253 = call-poly "Enqueue Message.vi"("error in (no error)"=w591, "Message Data"=w582, "Message"="InsertTextIntoDataFileNameFVIR", "Message Queue"=w589) -> ("error out"=w590:errorcluster)  [unwired: 6 in, 1 out]
      }
      frame "StartTestCaseLDO" {
        # "Reset the total flow and gas total\nSend latest timing parameters"
        # "Indicate that now a LDO test is active"
        # "Start - Enable/Disable buttons appropriately for an acquisition that has started, and update status display."
        n254 = call-poly "Enqueue Message.vi"("error in (no error)"=w683, "Message Data"="LDO test has started..." ("Acquiring and Logging..."), "Message"="Update Status - LDO", "Message Queue"=w689) -> ("error out"=w676:errorcluster, "dup Message Queue"=w673:refnum<queue>)  [unwired: 6 in]
        n255 = call "LDO_Setup_Parameters.vi"("Alicat_GasMeter"=w672, "Modbus"=w674, "error in (no error)"=w676, "UI in"=w673) -> ("error out"=w675:errorcluster)  [unwired: 7 in]
        n256 = call-poly "Enqueue Message.vi"("error in (no error)"=w675, "Message"="StartTestLDO", "Message Queue"=w674) -> ("error out"=w682:errorcluster)  [unwired: 7 in, 1 out]
        n257 = Bundle By Name(cluster=w680, "PLC Data Out.Data to Save.Test Case - LDO"="LDO_test" ("Acquiring and Logging...")) -> (w678:T2)
        n258 = Unbundle By Name(w678) -> ("PLC Data Out"=w677:T3)
        n259 = call-poly "Enqueue Message.vi"("error in (no error)"=w682, "Message Data"=w677, "Message"="InsertTextIntoDataFileNameLDO", "Message Queue"=w687) -> ("error out"=w688:errorcluster)  [unwired: 6 in, 1 out]
      }
      frame "StopTestCaseFVIR" {
        # "Start - Enable/Disable buttons appropriately for an acquisition that has started, and update status display."
        n260 = call-poly "Enqueue Message.vi"("error in (no error)"=w702, "Message"="StopTestFVIR", "Message Queue"=w703) -> ("error out"=w699:errorcluster)  [unwired: 7 in, 1 out]
        n261 = call-poly "Enqueue Message.vi"("error in (no error)"=w699, "Message Data"="Current FVIR test has stopped ..." ("Acquiring and Logging..."), "Message"="Update Status - FVIR", "Message Queue"=w700) -> ("error out"=w697:errorcluster)  [unwired: 6 in, 1 out]
      }
      frame "StopTestCaseFVIRLogFile" {
        # "Start - Enable/Disable buttons appropriately for an acquisition that has started, and update status display."
        n262 = call-poly "Enqueue Message.vi"("error in (no error)"=w714, "Message"="StopTestFVIR", "Message Queue"=w715) -> ("error out"=w711:errorcluster)  [unwired: 7 in, 1 out]
        n263 = call-poly "Enqueue Message.vi"("error in (no error)"=w711, "Message Data"="Current FVIR test has stopped ..." ("Acquiring and Logging..."), "Message"="Update Status - FVIR", "Message Queue"=w712) -> ("error out"=w709:errorcluster)  [unwired: 6 in, 1 out]
      }
      frame "StopTestCaseLDO" {
        # "Start - Enable/Disable buttons appropriately for an acquisition that has started, and update status display."
        n264 = call-poly "Enqueue Message.vi"("error in (no error)"=w726, "Message"="StopTestLDO", "Message Queue"=w727) -> ("error out"=w723:errorcluster)  [unwired: 7 in, 1 out]
        n265 = call-poly "Enqueue Message.vi"("error in (no error)"=w723, "Message Data"="Current LDO test has stopped ..." ("Acquiring and Logging..."), "Message"="Update Status - LDO", "Message Queue"=w724) -> ("error out"=w720:errorcluster)  [unwired: 6 in, 1 out]
      }
      frame "MannequinHomePos" {
        # "Start - Enable/Disable buttons appropriately for an acquisition that has started, and update status display."
        n266 = disable-structure shown="Disabled" {
          disable-tunnel: w733 -> [w741 _]
          frame Disabled {
            n267 = Unbundle By Name(w741) -> ("Stop Ref"=w746:refnum<vi>, "Start Ref"=w745:refnum<vi>, "Exit Ref"=w744:refnum<vi>)
            n268 = Build Array(w746) -> (w747:refnum<vi>[])
            n269 = Build Array(w745, w744) -> (w748:refnum<vi>[])
            n270 = call "Set Enable State on Multiple Controls.vi"("Enable?"=TRUE, "Controls"=w747) -> ()  [unwired: 10 in]
            n271 = call "Set Enable State on Multiple Controls.vi"("Enable?"=FALSE, "Controls"=w748) -> ()  [unwired: 10 in]
          }
          frame Enabled {
          }
        }
        n272 = call-poly "Enqueue Message.vi"("error in (no error)"=w735, "Message Data"="Operator clicked on: Move mannequin to Home Pos" ("Acquiring and Logging..."), "Message"="Update Status - FVIR", "Message Queue"=w732) -> ("error out"=w736:errorcluster)  [unwired: 6 in, 1 out]
        n273 = call-poly "Enqueue Message.vi"("error in (no error)"=w736, "Message"="MannequinGoToHomePos", "Message Queue"=w734) -> ("error out"=w738:errorcluster)  [unwired: 7 in, 1 out]
      }
      frame "MannequinWorkPos" {
        # "Start - Enable/Disable buttons appropriately for an acquisition that has started, and update status display."
        n274 = disable-structure shown="Disabled" {
          disable-tunnel: w753 -> [w761 _]
          frame Disabled {
            n275 = Unbundle By Name(w761) -> ("Stop Ref"=w766:refnum<vi>, "Start Ref"=w765:refnum<vi>, "Exit Ref"=w764:refnum<vi>)
            n276 = Build Array(w766) -> (w767:refnum<vi>[])
            n277 = Build Array(w765, w764) -> (w768:refnum<vi>[])
            n278 = call "Set Enable State on Multiple Controls.vi"("Enable?"=TRUE, "Controls"=w767) -> ()  [unwired: 10 in]
            n279 = call "Set Enable State on Multiple Controls.vi"("Enable?"=FALSE, "Controls"=w768) -> ()  [unwired: 10 in]
          }
          frame Enabled {
          }
        }
        n280 = call-poly "Enqueue Message.vi"("error in (no error)"=w755, "Message Data"="Operator clicked on: Move mannequin to Work Pos" ("Acquiring and Logging..."), "Message"="Update Status - FVIR", "Message Queue"=w752) -> ("error out"=w756:errorcluster)  [unwired: 6 in, 1 out]
        n281 = call-poly "Enqueue Message.vi"("error in (no error)"=w756, "Message"="MannequinGoToWorkPos", "Message Queue"=w754) -> ("error out"=w758:errorcluster)  [unwired: 7 in, 1 out]
      }
      frame "SpillCanHomePos" {
        # "Start - Enable/Disable buttons appropriately for an acquisition that has started, and update status display."
        n282 = disable-structure shown="Disabled" {
          disable-tunnel: w773 -> [w781 _]
          frame Disabled {
            n283 = Unbundle By Name(w781) -> ("Stop Ref"=w786:refnum<vi>, "Start Ref"=w785:refnum<vi>, "Exit Ref"=w784:refnum<vi>)
            n284 = Build Array(w786) -> (w787:refnum<vi>[])
            n285 = Build Array(w785, w784) -> (w788:refnum<vi>[])
            n286 = call "Set Enable State on Multiple Controls.vi"("Enable?"=TRUE, "Controls"=w787) -> ()  [unwired: 10 in]
            n287 = call "Set Enable State on Multiple Controls.vi"("Enable?"=FALSE, "Controls"=w788) -> ()  [unwired: 10 in]
          }
          frame Enabled {
          }
        }
        n288 = call-poly "Enqueue Message.vi"("error in (no error)"=w775, "Message Data"="Operator clicked on: Move gasoline can to Home Pos" ("Acquiring and Logging..."), "Message"="Update Status - FVIR", "Message Queue"=w772) -> ("error out"=w776:errorcluster)  [unwired: 6 in, 1 out]
        n289 = call-poly "Enqueue Message.vi"("error in (no error)"=w776, "Message"="SpillCanGoToHomePos", "Message Queue"=w774) -> ("error out"=w778:errorcluster)  [unwired: 7 in, 1 out]
      }
      frame "SpillCanWorkPos" {
        # "Start - Enable/Disable buttons appropriately for an acquisition that has started, and update status display."
        n290 = disable-structure shown="Disabled" {
          disable-tunnel: w793 -> [w801 _]
          frame Disabled {
            n291 = Unbundle By Name(w801) -> ("Stop Ref"=w806:refnum<vi>, "Start Ref"=w805:refnum<vi>, "Exit Ref"=w804:refnum<vi>)
            n292 = Build Array(w806) -> (w807:refnum<vi>[])
            n293 = Build Array(w805, w804) -> (w808:refnum<vi>[])
            n294 = call "Set Enable State on Multiple Controls.vi"("Enable?"=TRUE, "Controls"=w807) -> ()  [unwired: 10 in]
            n295 = call "Set Enable State on Multiple Controls.vi"("Enable?"=FALSE, "Controls"=w808) -> ()  [unwired: 10 in]
          }
          frame Enabled {
          }
        }
        n296 = call-poly "Enqueue Message.vi"("error in (no error)"=w795, "Message Data"="Operator clicked on: Move gasoline can to Work Pos" ("Acquiring and Logging..."), "Message"="Update Status - FVIR", "Message Queue"=w792) -> ("error out"=w796:errorcluster)  [unwired: 6 in, 1 out]
        n297 = call-poly "Enqueue Message.vi"("error in (no error)"=w796, "Message"="SpillCanGoToWorkPos", "Message Queue"=w794) -> ("error out"=w798:errorcluster)  [unwired: 7 in, 1 out]
      }
      frame "WaterOutletOpenFVIR" {
        # "Start - Enable/Disable buttons appropriately for an acquisition that has started, and update status display."
        n298 = call-poly "Enqueue Message.vi"("error in (no error)"=w817, "Message Data"="Operator clicked on: Water Outlet Valve Open FVIR" ("Acquiring and Logging..."), "Message"="Update Status - FVIR", "Message Queue"=w816) -> ("error out"=w818:errorcluster)  [unwired: 6 in, 1 out]
        n299 = call-poly "Enqueue Message.vi"("error in (no error)"=w818, "Message"="WaterOutletOpenFVIR", "Message Queue"=w815) -> ("error out"=w819:errorcluster)  [unwired: 7 in, 1 out]
      }
      frame "WaterOutletOpenLDO" {
        # "Start - Enable/Disable buttons appropriately for an acquisition that has started, and update status display."
        n300 = call-poly "Enqueue Message.vi"("error in (no error)"=w829, "Message Data"="Operator clicked on: Water Outlet Valve Open LDO" ("Acquiring and Logging..."), "Message"="Update Status - LDO", "Message Queue"=w828) -> ("error out"=w830:errorcluster)  [unwired: 6 in, 1 out]
        n301 = call-poly "Enqueue Message.vi"("error in (no error)"=w830, "Message"="WaterOutletOpenLDO", "Message Queue"=w827) -> ("error out"=w831:errorcluster)  [unwired: 7 in, 1 out]
      }
      frame "WaterOutletCloseFVIR" {
        # "Start - Enable/Disable buttons appropriately for an acquisition that has started, and update status display."
        n302 = call-poly "Enqueue Message.vi"("error in (no error)"=w841, "Message Data"="Operator clicked on: Water Outlet Valve Close FVIR" ("Acquiring and Logging..."), "Message"="Update Status - FVIR", "Message Queue"=w840) -> ("error out"=w842:errorcluster)  [unwired: 6 in, 1 out]
        n303 = call-poly "Enqueue Message.vi"("error in (no error)"=w842, "Message"="WaterOutletCloseFVIR", "Message Queue"=w839) -> ("error out"=w843:errorcluster)  [unwired: 7 in, 1 out]
      }
      frame "WaterOutletCloseLDO" {
        # "Start - Enable/Disable buttons appropriately for an acquisition that has started, and update status display."
        n304 = call-poly "Enqueue Message.vi"("error in (no error)"=w853, "Message Data"="Operator clicked on: Water Outlet Valve Close LDO" ("Acquiring and Logging..."), "Message"="Update Status - LDO", "Message Queue"=w852) -> ("error out"=w854:errorcluster)  [unwired: 6 in, 1 out]
        n305 = call-poly "Enqueue Message.vi"("error in (no error)"=w854, "Message"="WaterOutletCloseLDO", "Message Queue"=w851) -> ("error out"=w855:errorcluster)  [unwired: 7 in, 1 out]
      }
      frame "WaterInletOpenFVIR" {
        # "Start - Enable/Disable buttons appropriately for an acquisition that has started, and update status display."
        n306 = call-poly "Enqueue Message.vi"("error in (no error)"=w865, "Message Data"="Operator clicked on: Water Inlet Valve Open FVIR" ("Acquiring and Logging..."), "Message"="Update Status - FVIR", "Message Queue"=w864) -> ("error out"=w866:errorcluster)  [unwired: 6 in, 1 out]
        n307 = call-poly "Enqueue Message.vi"("error in (no error)"=w866, "Message"="WaterInletOpenFVIR", "Message Queue"=w863) -> ("error out"=w867:errorcluster)  [unwired: 7 in, 1 out]
      }
      frame "WaterInletOpenLDO" {
        # "Start - Enable/Disable buttons appropriately for an acquisition that has started, and update status display."
        n308 = call-poly "Enqueue Message.vi"("error in (no error)"=w877, "Message Data"="Operator clicked on: Water Inlet Valve Open LDO" ("Acquiring and Logging..."), "Message"="Update Status - LDO", "Message Queue"=w876) -> ("error out"=w878:errorcluster)  [unwired: 6 in, 1 out]
        n309 = call-poly "Enqueue Message.vi"("error in (no error)"=w878, "Message"="WaterInletOpenLDO", "Message Queue"=w875) -> ("error out"=w879:errorcluster)  [unwired: 7 in, 1 out]
      }
      frame "WaterInletCloseFVIR" {
        # "Start - Enable/Disable buttons appropriately for an acquisition that has started, and update status display."
        n310 = call-poly "Enqueue Message.vi"("error in (no error)"=w889, "Message Data"="Operator clicked on: Water Inlet Valve Close FVIR" ("Acquiring and Logging..."), "Message"="Update Status - FVIR", "Message Queue"=w888) -> ("error out"=w890:errorcluster)  [unwired: 6 in, 1 out]
        n311 = call-poly "Enqueue Message.vi"("error in (no error)"=w890, "Message"="WaterInletCloseFVIR", "Message Queue"=w887) -> ("error out"=w891:errorcluster)  [unwired: 7 in, 1 out]
      }
      frame "WaterInletCloseLDO" {
        # "Start - Enable/Disable buttons appropriately for an acquisition that has started, and update status display."
        n312 = call-poly "Enqueue Message.vi"("error in (no error)"=w901, "Message Data"="Operator clicked on: Water Inlet Valve Close LDO" ("Acquiring and Logging..."), "Message"="Update Status - LDO", "Message Queue"=w900) -> ("error out"=w902:errorcluster)  [unwired: 6 in, 1 out]
        n313 = call-poly "Enqueue Message.vi"("error in (no error)"=w902, "Message"="WaterInletCloseLDO", "Message Queue"=w899) -> ("error out"=w903:errorcluster)  [unwired: 7 in, 1 out]
      }
      frame "GasSolenoidOpenFVIR" {
        # "Start - Enable/Disable buttons appropriately for an acquisition that has started, and update status display."
        n314 = call-poly "Enqueue Message.vi"("error in (no error)"=w913, "Message Data"="Operator clicked on: Gas Solenoid Valve Open FVIR" ("Acquiring and Logging..."), "Message"="Update Status - FVIR", "Message Queue"=w912) -> ("error out"=w914:errorcluster)  [unwired: 6 in, 1 out]
        n315 = call-poly "Enqueue Message.vi"("error in (no error)"=w914, "Message"="GasSolenoidOpenFVIR", "Message Queue"=w911) -> ("error out"=w915:errorcluster)  [unwired: 7 in, 1 out]
      }
      frame "GasSolenoidOpenLDO" {
        # "Start - Enable/Disable buttons appropriately for an acquisition that has started, and update status display."
        n316 = call-poly "Enqueue Message.vi"("error in (no error)"=w925, "Message Data"="Operator clicked on: Gas Solenoid Valve Open LDO" ("Acquiring and Logging..."), "Message"="Update Status - LDO", "Message Queue"=w924) -> ("error out"=w926:errorcluster)  [unwired: 6 in, 1 out]
        n317 = call-poly "Enqueue Message.vi"("error in (no error)"=w926, "Message"="GasSolenoidOpenLDO", "Message Queue"=w923) -> ("error out"=w927:errorcluster)  [unwired: 7 in, 1 out]
      }
      frame "GasSolenoidCloseFVIR" {
        # "Start - Enable/Disable buttons appropriately for an acquisition that has started, and update status display."
        n318 = call-poly "Enqueue Message.vi"("error in (no error)"=w937, "Message Data"="Operator clicked on: Gas Solenoid Valve Close FVIR" ("Acquiring and Logging..."), "Message"="Update Status - FVIR", "Message Queue"=w936) -> ("error out"=w938:errorcluster)  [unwired: 6 in, 1 out]
        n319 = call-poly "Enqueue Message.vi"("error in (no error)"=w938, "Message"="GasSolenoidCloseFVIR", "Message Queue"=w935) -> ("error out"=w939:errorcluster)  [unwired: 7 in, 1 out]
      }
      frame "GasSolenoidCloseLDO" {
        # "Start - Enable/Disable buttons appropriately for an acquisition that has started, and update status display."
        n320 = call-poly "Enqueue Message.vi"("error in (no error)"=w949, "Message Data"="Operator clicked on: Gas Solenoid Valve Close LDO" ("Acquiring and Logging..."), "Message"="Update Status - LDO", "Message Queue"=w948) -> ("error out"=w950:errorcluster)  [unwired: 6 in, 1 out]
        n321 = call-poly "Enqueue Message.vi"("error in (no error)"=w950, "Message"="GasSolenoidCloseLDO", "Message Queue"=w947) -> ("error out"=w951:errorcluster)  [unwired: 7 in, 1 out]
      }
      frame "WaterFlowOpenFVIR" {
        # "Start - Enable/Disable buttons appropriately for an acquisition that has started, and update status display."
        n322 = call-poly "Enqueue Message.vi"("error in (no error)"=w961, "Message Data"="Operator clicked on: Water Flow Intellifaucet DRK375 Open FVIR" ("Acquiring and Logging..."), "Message"="Update Status - FVIR", "Message Queue"=w960) -> ("error out"=w962:errorcluster)  [unwired: 6 in, 1 out]
        n323 = call-poly "Enqueue Message.vi"("error in (no error)"=w962, "Message"="WaterFlowOpenFVIR", "Message Queue"=w959) -> ("error out"=w963:errorcluster)  [unwired: 7 in, 1 out]
      }
      frame "WaterFlowStartLDO" {
        # "Start - Enable/Disable buttons appropriately for an acquisition that has started, and update status display."
        n324 = call-poly "Enqueue Message.vi"("error in (no error)"=w973, "Message Data"="Operator clicked on: Water Flow Intellifaucet DRK375 Start" ("Acquiring and Logging..."), "Message"="Update Status - LDO", "Message Queue"=w972) -> ("error out"=w974:errorcluster)  [unwired: 6 in, 1 out]
        n325 = call-poly "Enqueue Message.vi"("error in (no error)"=w974, "Message"="WaterFlowStartLDO", "Message Queue"=w971) -> ("error out"=w975:errorcluster)  [unwired: 7 in, 1 out]
      }
      frame "WaterFlowCloseFVIR" {
        # "Start - Enable/Disable buttons appropriately for an acquisition that has started, and update status display."
        n326 = call-poly "Enqueue Message.vi"("error in (no error)"=w985, "Message Data"="Operator clicked on: Water Flow Intellifaucet DRK375 Close FVIR" ("Acquiring and Logging..."), "Message"="Update Status - FVIR", "Message Queue"=w984) -> ("error out"=w986:errorcluster)  [unwired: 6 in, 1 out]
        n327 = call-poly "Enqueue Message.vi"("error in (no error)"=w986, "Message"="WaterFlowCloseFVIR", "Message Queue"=w983) -> ("error out"=w987:errorcluster)  [unwired: 7 in, 1 out]
      }
      frame "WaterFlowStartZeroLDO" {
        # "Start - Enable/Disable buttons appropriately for an acquisition that has started, and update status display."
        n328 = call-poly "Enqueue Message.vi"("error in (no error)"=w997, "Message Data"="Operator clicked on: Water Flow Intellifaucet DRK375 Start" ("Acquiring and Logging..."), "Message"="Update Status - LDO", "Message Queue"=w996) -> ("error out"=w998:errorcluster)  [unwired: 6 in, 1 out]
        n329 = call-poly "Enqueue Message.vi"("error in (no error)"=w998, "Message"="WaterFlowStartZeroLDO", "Message Queue"=w995) -> ("error out"=w999:errorcluster)  [unwired: 7 in, 1 out]
      }
      frame "WaterFlowPropOpenFVIR" {
        # "Start - Enable/Disable buttons appropriately for an acquisition that has started, and update status display."
        n330 = call-poly "Enqueue Message.vi"("error in (no error)"=w1009, "Message Data"="Operator clicked on: Water Outlet Flow Proportional EPV-312B Open FVIR" ("Acquiring and Logging..."), "Message"="Update Status - FVIR", "Message Queue"=w1008) -> ("error out"=w1010:errorcluster)  [unwired: 6 in, 1 out]
        n331 = call-poly "Enqueue Message.vi"("error in (no error)"=w1010, "Message"="WaterFlowPropOpenFVIR", "Message Queue"=w1007) -> ("error out"=w1011:errorcluster)  [unwired: 7 in, 1 out]
      }
      frame "WaterFlowPropOpenLDO" {
        # "Start - Enable/Disable buttons appropriately for an acquisition that has started, and update status display."
        n332 = call-poly "Enqueue Message.vi"("error in (no error)"=w1021, "Message Data"="Operator clicked on: Water Outlet Flow Proportional EPV-312B Open LDO" ("Acquiring and Logging..."), "Message"="Update Status - LDO", "Message Queue"=w1020) -> ("error out"=w1022:errorcluster)  [unwired: 6 in, 1 out]
        n333 = call-poly "Enqueue Message.vi"("error in (no error)"=w1022, "Message"="WaterFlowPropOpenLDO", "Message Queue"=w1019) -> ("error out"=w1023:errorcluster)  [unwired: 7 in, 1 out]
      }
      frame "WaterFlowPropCloseFVIR" {
        # "Start - Enable/Disable buttons appropriately for an acquisition that has started, and update status display."
        n334 = call-poly "Enqueue Message.vi"("error in (no error)"=w1033, "Message Data"="Operator clicked on: Water Outlet Flow Proportional EPV-312B Close FVIR" ("Acquiring and Logging..."), "Message"="Update Status - FVIR", "Message Queue"=w1032) -> ("error out"=w1034:errorcluster)  [unwired: 6 in, 1 out]
        n335 = call-poly "Enqueue Message.vi"("error in (no error)"=w1034, "Message"="WaterFlowPropCloseFVIR", "Message Queue"=w1031) -> ("error out"=w1035:errorcluster)  [unwired: 7 in, 1 out]
      }
      frame "WaterFlowPropCloseLDO" {
        # "Start - Enable/Disable buttons appropriately for an acquisition that has started, and update status display."
        n336 = call-poly "Enqueue Message.vi"("error in (no error)"=w1045, "Message Data"="Operator clicked on: Water Outlet Flow Proportional EPV-312B Close LDO" ("Acquiring and Logging..."), "Message"="Update Status - LDO", "Message Queue"=w1044) -> ("error out"=w1046:errorcluster)  [unwired: 6 in, 1 out]
        n337 = call-poly "Enqueue Message.vi"("error in (no error)"=w1046, "Message"="WaterFlowPropCloseLDO", "Message Queue"=w1043) -> ("error out"=w1047:errorcluster)  [unwired: 7 in, 1 out]
      }
      frame "WaterFlowStopLDO" {
        n338 = call-poly "Enqueue Message.vi"("error in (no error)"=w1054, "Message Data"="Operator clicked on: Water Flow Intellifaucet DRK375 Stop" ("Acquiring and Logging..."), "Message"="Update Status - LDO", "Message Queue"=w1051) -> ("error out"=w1058:errorcluster)  [unwired: 6 in, 1 out]
        n339 = call-poly "Enqueue Message.vi"("error in (no error)"=w1058, "Message"="WaterFlowStopLDO", "Message Queue"=w1052) -> ("error out"=w1053:errorcluster)  [unwired: 7 in, 1 out]
      }
      frame "WaterFlowStopZeroLDO" {
        n340 = call-poly "Enqueue Message.vi"("error in (no error)"=w1066, "Message Data"="Operator clicked on: Water Flow Intellifaucet DRK375 Stop" ("Acquiring and Logging..."), "Message"="Update Status - LDO", "Message Queue"=w1063) -> ("error out"=w1070:errorcluster)  [unwired: 6 in, 1 out]
        n341 = call-poly "Enqueue Message.vi"("error in (no error)"=w1070, "Message"="WaterFlowStopZeroLDO", "Message Queue"=w1064) -> ("error out"=w1065:errorcluster)  [unwired: 7 in, 1 out]
      }
      frame "OilSpray08Open" {
        # "Start - Enable/Disable buttons appropriately for an acquisition that has started, and update status display."
        n342 = call-poly "Enqueue Message.vi"("error in (no error)"=w1081, "Message Data"="Operator clicked on: Oil Spray 0.8 cc/min Open" ("Acquiring and Logging..."), "Message"="Update Status - LDO", "Message Queue"=w1080) -> ("error out"=w1082:errorcluster)  [unwired: 6 in, 1 out]
        n343 = call-poly "Enqueue Message.vi"("error in (no error)"=w1082, "Message"="OilSpray08Open", "Message Queue"=w1075) -> ("error out"=w1083:errorcluster)  [unwired: 7 in, 1 out]
      }
      frame "OilSpray08Close" {
        # "Start - Enable/Disable buttons appropriately for an acquisition that has started, and update status display."
        n344 = call-poly "Enqueue Message.vi"("error in (no error)"=w1093, "Message Data"="Operator clicked on: Oil Spray 0.8 cc/min Close" ("Acquiring and Logging..."), "Message"="Update Status - LDO", "Message Queue"=w1092) -> ("error out"=w1094:errorcluster)  [unwired: 6 in, 1 out]
        n345 = call-poly "Enqueue Message.vi"("error in (no error)"=w1094, "Message"="OilSpray08Close", "Message Queue"=w1087) -> ("error out"=w1095:errorcluster)  [unwired: 7 in, 1 out]
      }
      frame "OilSpray11Open" {
        # "Start - Enable/Disable buttons appropriately for an acquisition that has started, and update status display."
        n346 = call-poly "Enqueue Message.vi"("error in (no error)"=w1105, "Message Data"="Operator clicked on: Oil Spray 1.1 cc/min Open" ("Acquiring and Logging..."), "Message"="Update Status - LDO", "Message Queue"=w1104) -> ("error out"=w1106:errorcluster)  [unwired: 6 in, 1 out]
        n347 = call-poly "Enqueue Message.vi"("error in (no error)"=w1106, "Message"="OilSpray11Open", "Message Queue"=w1099) -> ("error out"=w1107:errorcluster)  [unwired: 7 in, 1 out]
      }
      frame "OilSpray11Close" {
        # "Start - Enable/Disable buttons appropriately for an acquisition that has started, and update status display."
        n348 = call-poly "Enqueue Message.vi"("error in (no error)"=w1117, "Message Data"="Operator clicked on: Oil Spray 1.1 cc/min Close" ("Acquiring and Logging..."), "Message"="Update Status - LDO", "Message Queue"=w1116) -> ("error out"=w1118:errorcluster)  [unwired: 6 in, 1 out]
        n349 = call-poly "Enqueue Message.vi"("error in (no error)"=w1118, "Message"="OilSpray11Close", "Message Queue"=w1111) -> ("error out"=w1119:errorcluster)  [unwired: 7 in, 1 out]
      }
      frame "OilSpray133Open" {
        # "Not used right now."
        # "Start - Enable/Disable buttons appropriately for an acquisition that has started, and update status display."
        n350 = call-poly "Enqueue Message.vi"("error in (no error)"=w1129, "Message Data"="Operator clicked on: Oil Spray 1.33 cc/min Open" ("Acquiring and Logging..."), "Message"="Update Status - LDO", "Message Queue"=w1128) -> ("error out"=w1130:errorcluster)  [unwired: 6 in, 1 out]
        n351 = call-poly "Enqueue Message.vi"("error in (no error)"=w1130, "Message"="OilSpray133Open", "Message Queue"=w1123) -> ("error out"=w1131:errorcluster)  [unwired: 7 in, 1 out]
      }
      frame "OilSpray133Close" {
        # "Start - Enable/Disable buttons appropriately for an acquisition that has started, and update status display."
        n352 = call-poly "Enqueue Message.vi"("error in (no error)"=w1141, "Message Data"="Operator clicked on: Oil Spray 1.33 cc/min Close" ("Acquiring and Logging..."), "Message"="Update Status - LDO", "Message Queue"=w1140) -> ("error out"=w1142:errorcluster)  [unwired: 6 in, 1 out]
        n353 = call-poly "Enqueue Message.vi"("error in (no error)"=w1142, "Message"="OilSpray133Close", "Message Queue"=w1135) -> ("error out"=w1143:errorcluster)  [unwired: 7 in, 1 out]
      }
      frame "HeaterON" {
        # "Start - Enable/Disable buttons appropriately for an acquisition that has started, and update status display."
        n354 = call-poly "Enqueue Message.vi"("error in (no error)"=w1153, "Message Data"="Operator clicked on: Heater ON..." ("Acquiring and Logging..."), "Message"="Update Status - LDO", "Message Queue"=w1152) -> ("error out"=w1154:errorcluster)  [unwired: 6 in, 1 out]
        n355 = call-poly "Enqueue Message.vi"("error in (no error)"=w1154, "Message"="HeaterON", "Message Queue"=w1151) -> ("error out"=w1155:errorcluster)  [unwired: 7 in, 1 out]
      }
      frame "HeaterOFF" {
        # "Start - Enable/Disable buttons appropriately for an acquisition that has started, and update status display."
        n356 = call-poly "Enqueue Message.vi"("error in (no error)"=w1165, "Message Data"="Operator clicked on: Heater OFF..." ("Acquiring and Logging..."), "Message"="Update Status - LDO", "Message Queue"=w1164) -> ("error out"=w1166:errorcluster)  [unwired: 6 in, 1 out]
        n357 = call-poly "Enqueue Message.vi"("error in (no error)"=w1166, "Message"="HeaterOFF", "Message Queue"=w1163) -> ("error out"=w1167:errorcluster)  [unwired: 7 in, 1 out]
      }
      frame "ConveyorON" {
        n358 = call-poly "Enqueue Message.vi"("error in (no error)"=w1174, "Message Data"="Operator clicked on: Conveyor ON..." ("Acquiring and Logging..."), "Message"="Update Status - LDO", "Message Queue"=w1171) -> ("error out"=w1178:errorcluster)  [unwired: 6 in, 1 out]
        n359 = call-poly "Enqueue Message.vi"("error in (no error)"=w1178, "Message"="ConveyorON", "Message Queue"=w1172) -> ("error out"=w1173:errorcluster)  [unwired: 7 in, 1 out]
      }
      frame "ConveyorOFF" {
        n360 = call-poly "Enqueue Message.vi"("error in (no error)"=w1186, "Message Data"="Operator clicked on: Conveyor OFF..." ("Acquiring and Logging..."), "Message"="Update Status - LDO", "Message Queue"=w1182) -> ("error out"=w1190:errorcluster)  [unwired: 6 in, 1 out]
        n361 = call-poly "Enqueue Message.vi"("error in (no error)"=w1190, "Message"="ConveyorOFF", "Message Queue"=w1181) -> ("error out"=w1185:errorcluster)  [unwired: 7 in, 1 out]
      }
      frame "BlowerON" {
        n362 = call-poly "Enqueue Message.vi"("error in (no error)"=w1198, "Message Data"="Operator clicked on: Blower ON..." ("Acquiring and Logging..."), "Message"="Update Status - LDO", "Message Queue"=w1196) -> ("error out"=w1202:errorcluster)  [unwired: 6 in, 1 out]
        n363 = call-poly "Enqueue Message.vi"("error in (no error)"=w1202, "Message"="BlowerON", "Message Queue"=w1195) -> ("error out"=w1197:errorcluster)  [unwired: 7 in, 1 out]
      }
      frame "BlowerOFF" {
        n364 = call-poly "Enqueue Message.vi"("error in (no error)"=w1210, "Message Data"="Operator clicked on: Conveyor OFF..." ("Acquiring and Logging..."), "Message"="Update Status - LDO", "Message Queue"=w1208) -> ("error out"=w1214:errorcluster)  [unwired: 6 in, 1 out]
        n365 = call-poly "Enqueue Message.vi"("error in (no error)"=w1214, "Message"="BlowerOFF", "Message Queue"=w1207) -> ("error out"=w1209:errorcluster)  [unwired: 7 in, 1 out]
      }
      frame "SendParamToPLCFVIR" {
        # "Start - Enable/Disable buttons appropriately for an acquisition that has started, and update status display."
        n366 = call-poly "Enqueue Message.vi"("error in (no error)"=w1231, "Message Data"="Operator clicked on: Send parameters to PLC FVIR ..." ("Acquiring and Logging..."), "Message"="Update Status - FVIR", "Message Queue"=w1230) -> ("error out"=w1232:errorcluster)  [unwired: 6 in, 1 out]
        n367 = Build Array("Time Delay of Change direction of Mannequin Actuators", "Number of Mannequin Movement", "Water Outlet Proportional Valve EPV-312B", "Water Temperature Intellifaucet DRK375", "Water Flow Intellifaucet DRK375", "Time Pause Between Next Mannequin Sequence") -> (w1221:u16[])
        n368 = call-poly "Enqueue Message.vi"("error in (no error)"=w1232, "Message Data"=w1221, "Message"="SendParamToPLCFVIR", "Message Queue"=w1229) -> ("error out"=w1233:errorcluster)  [unwired: 6 in, 1 out]
      }
      frame "SendParamToPLCLDO" {
        # "Start - Enable/Disable buttons appropriately for an acquisition that has started, and update status display."
        n369 = call-poly "Enqueue Message.vi"("error in (no error)"=w1261, "Message Data"="Operator clicked on: Send parameters to PLC LDO ..." ("Acquiring and Logging..."), "Message"="Update Status - LDO", "Message Queue"=w1260) -> ("error out"=w1262:errorcluster)  [unwired: 6 in, 1 out]
        n370 = Build Array("Burner cycle 1 to 10 - Duty cycle ON (default 55 min.)", "Burner cycle 1 to 10 - Duty cycle OFF (default 5 min.)", "Burner cycle 11 to 12 - Duty cycle ON (default 235 min.)", "Burner cycle 11 to 12 - Duty cycle OFF (default 5 min.)", "Burner cycle 13 to end - Duty cycle ON (default 55 min.)", "Burner cycle 13 to end - Duty cycle OFF (default 5 min.)", "Oil 1st sequence ON (default 5 min.)", "Oil 1st sequence OFF (default 5 min.)", "All subsequent sequence ON (default 3 min.)", "All subsequent sequence OFF (default 27 min.)", "Oil spray preconditioning period ON (default 10 min.)", "Oil spray preconditioning period OFF  (default 20 min.)", "Precondition Purge Gallons") -> (w1258:u16[])
        n371 = call-poly "Enqueue Message.vi"("error in (no error)"=w1262, "Message Data"=w1258, "Message"="SendParamToPLCLDO", "Message Queue"=w1238) -> ("error out"=w1240:errorcluster)  [unwired: 6 in, 1 out]
        n372 = local read "Temp (°F) - Automatic Mode"() -> (w1237:dbl)
        n373 = local read "Valve % Open - Automatic Mode"() -> (w1236:dbl)
        n374 = call "LDO_Update_Intellifaucet_Parameters.vi"("error in (no error)"=w1240, "Valve % Open - Automatic Mode"=w1236, "Temp (°F) - Automatic Mode"=w1237, "Modbus Input"=w1238) -> ("error out"=w1239:errorcluster)  [unwired: 7 in]
      }
      frame "DataToShow" {
        # "FVIR block sends out boolean if one of the 4 tubes are >= 1.8"
        # "If one of the 4 tubes for % Butane are >= 1.8, the test will stop"
        # "Update Status - Convert the message data to a string to display in the Status indicator."
        n375 = Variant To Data(error in=w1278, type=string[] [], Variant=w1277) -> (data=w1273:string[], error out=w1272:errorcluster)
        n376 = call "DisplayTemperaturesFVIR.vi"("Array"=w1273) -> ("FVIR array 2"=→"Temperatures - FVIR":string[][], "Logical OR array"=w1268:bool)  [unwired: 8 in]
        n377 = case shown="True" w1268 {
          tunnel: w1272 -> [w1281 w1286]
          tunnel: [w1281 w1285] -> w1271
          tunnel: w1270 -> [_ w1284]
          tunnel: w1269 -> [w1280 w1283]
          tunnel: [w1280 w1282] -> w1267
          frame False {
          }
          frame True {
            n378 = case shown="False" w1283 {
              tunnel: w1286 -> [w1288 w1293]
              tunnel: [w1288 w1292] -> w1285
              tunnel: w1284 -> [_ w1291]
              tunnel: [TRUE ("new element/subarray") TRUE ("new element/subarray")] -> w1282
              frame True {
              }
              frame False {
                n379 = call-poly "Enqueue Message.vi"("error in (no error)"=w1293, "Message"="StopTestCaseFVIR", "Message Queue"=w1291) -> ("error out"=w1292:errorcluster)  [unwired: 7 in, 1 out]
              }
            }
          }
        }
        "Higher than 1.8% butane" <- w1267
        n380 = Merge Errors(w1271) -> (w1279:errorcluster)
      }
      frame "DisplayAllData" {
        n381 = Unbundle By Name(w1314) -> ("PLC Data Out"=w1323:T3)
        n382 = Unbundle By Name(w1314) -> ("PLC Data Out"=w1313:T3, "Gas Data"=w1312:T7, "Inficon Data Input"=w1311:T10, "Ultramat 23"=w1317:string[][], "PLC Data Out.LDO Control Input.Test chamber is in sequence - LDO"=w1299:bool, "PLC Data Out.LDO Control Input.Start recording data - LDO"=w1298:bool)
        n383 = Unbundle By Name(w1323) -> ("FVIR Data Input.FVIR PLC lifebit"=→"FVIR PLC lifebit":bool, "FVIR Data Input.Mannequin is moving - FVIR"=→"Mannequin is moving - FVIR":bool, "FVIR Data Input.Can is spilling - FVIR"=→"Can is spilling - FVIR":bool, "FVIR Data Input.Water Outlet Valve - FVIR"=→"Water Outlet Valve - FVIR":bool, "FVIR Data Input.Water Inlet Valve - FVIR"=→"Water Inlet Valve - FVIR":bool, "FVIR Data Input.Gas Solenoid Valve - FVIR"=→"Gas Solenoid Valuce - FVIR":bool, "FVIR Data Input.Water flow DRK375 is open - FVIR"=→"Water flow DRK375 is open - FVIR":bool, "FVIR Data Input.Actuator mannequin is going to Home Pos - FVIR"=→"Actuator mannequin is going to Home Pos - FVIR":bool, "FVIR Data Input.Actuator mannequin is going to Work Pos - FVIR"=→"Actuator mannequin is going to Work Pos - FVIR":bool, "FVIR Data Input.Actuator spill can is going to Home Pos - FVIR"=→"Actuator spill can is going to Home Pos - FVIR":bool, "FVIR Data Input.Actuator spill can is going to Work Pos - FVIR"=→"Actuator spill can is going to Work Pos - FVIR":bool, "FVIR Data Input.Start recording data - FVIR"=→"Start recording data - FVIR":bool, "FVIR Data Input.Status for Error - FVIR"=→"Status for error - FVIR":string, "FVIR Data Input.Error-FVIR"=→"Error - FVIR":bool, "FVIR Data Input.Sensors -FVIR"=→"Sensors - FVIR":string[][], "FVIR Data Input.Water Outlet Flow Proportional - FVIR"=→"Water Outlet Flow Proportional - FVIR":bool, "FVIR Data Input.Test chamber is in sequence - FVIR"=→"Test chamber is in sequence - FVIR":bool)
        n384 = Unbundle By Name(w1323) -> ("LDO Control Input.Start recording data - LDO"=→"Start recording data - LDO":bool, "LDO Control Input.Water Outlet Valve - LDO"=→"Water Outlet Valve":bool, "LDO Control Input.Water Inlet Valve - LDO"=→"Water Inlet Valve":bool, "LDO Control Input.Gas Solenoid Valve - LDO"=→"Gas Solenoid Valve":bool, "LDO Control Input.Water flow DRK375 is open - LDO"=→"Intellifaucet Start":bool, "LDO Control Input.Oil spray 0.8cc/min - LDO"=→"Oil spray 0.8cc/min":bool, "LDO Control Input.Oil spray 1.1cc/min - LDO"=→"Oil spray 1.1cc/min":bool, "LDO Control Input.Oil spray 1.33cc/min - LDO"=→"Oil spray 1.33cc/min":bool, "LDO Control Input.Rotary Actuator (ON/OFF) - LDO"=→"Rotary Actuator (ON/OFF)":bool, "LDO Control Input.Water Outlet Flow Proportional - LDO"=→"Water Outlet Flow Proportional":bool, "LDO Control Input.Status for error - LDO"=→"Status for error - LDO":string, "LDO Control Input.Error - LDO"=→"Error - LDO":bool, "LDO Control Input.Test chamber is in sequence - LDO"=→"Test chamber is in sequence":bool, "LDO Control Input.Conveyor ON/OFF"=→"Conveyor":bool, "LDO Control Input.Blower ON/OFF"=→"Blower":bool)
        n385 = control-ref of="Start recording data - LDO"() -> (w1294:refnum<vi>)
        n386 = control-ref of="Oil spray 1.33cc/min"() -> (w1304:refnum<vi>)
        n387 = control-ref of="Oil spray 1.1cc/min"() -> (w1306:refnum<vi>)
        n388 = control-ref of="Oil spray 0.8cc/min"() -> (w1307:refnum<vi>)
        n389 = control-ref of="Burner"() -> (w1308:refnum<vi>)
        n390 = call "LDO Array Data.vi"("PLC Data In"=w1313, "Burner ON Ref"=w1308, "0.8 ML Ref"=w1307, "1.1 ML Ref"=w1306, "Gas Data"=w1312, "Inficon Data Input"=w1311, "1.33 ML Ref"=w1304, "Ultramat 23"=w1317, "Start recording data"=w1294, "error in (no error)"=w1322, "Event Booleans in"=w1309, "Pilot Rate (BTU/hr)"="Pilot Rate (BTU/hr)") -> ("PLC Data Out"=w1303:T3, "LDO Array"=w1305:string[][], "Event Booleans out"=w1296:T1, "error out"=w1302:errorcluster)
        "Data" <- w1305
        n391 = And(x=w1299, y=w1298) -> (x .and. y?=w1297:bool)
        n392 = case shown="True" w1297 {
          tunnel: w1302 -> [w1353 w1356]
          tunnel: [w1353 w1355] -> w1301
          tunnel: w1300 -> [_ w1354]
          frame False {
          }
          frame True {
            n393 = call-poly "Enqueue Message.vi"("error in (no error)"=w1356, "Message"="LDOUpdateFlowTarget", "Message Queue"=w1354) -> ("error out"=w1355:errorcluster)  [unwired: 7 in, 1 out]
          }
        }
        n394 = Unbundle By Name(w1296) -> ("Burner ON"=→"Burner":bool)
        n395 = Bundle By Name(cluster=w1314, "PLC Data Out"=w1303, "PLC Data Out.Data to Save.LDO Full Data"=w1305) -> (w1318:T2)
      }
      frame "LDOUpdateFlowTarget" {
        n396 = Unbundle By Name(w1358) -> ("PLC Data Out.LDO Control Input.Thermal Efficiency Rate (GPM)"=w1363:dbl, "PLC Data Out.LDO Control Input.Totalized Flow (Gallons)"=w1362:dbl)
        n397 = Greater?(x=w1362, y="Start Auto GPM Gallons") -> (0:w1360:bool)
        n398 = case shown="True" w1360 {
          tunnel: w1366 -> [w1370 w1376]
          tunnel: w1365 -> [w1372 w1373]
          tunnel: [w1371 w1375] -> w1364
          tunnel: w1363 -> [_ w1374]
          frame False {
            n399 = call "Update_Flow_Target.vi"("error in"=w1372, "Output Flow Rate Target (Automated Test)"=0.76, "Modbus"=w1370) -> ("error out"=w1371:errorcluster)  [unwired: 8 in]
          }
          frame True {
            n400 = call "Update_Flow_Target.vi"("error in"=w1373, "Output Flow Rate Target (Automated Test)"=w1374, "Modbus"=w1376) -> ("error out"=w1375:errorcluster)  [unwired: 8 in]
          }
        }
      }
      frame "DisplayValuesFromPLC" {
        # "Update Status - Convert the message data to a string to display in the Status indicator."
        n401 = Unbundle By Name(w1380) -> ("PLC Data Out"=w1381:T3)
        n402 = Variant To Data(error in=w1400, type=u16[] [1, 0, 0, 0, 0, 0, 0, 0] ("Input Registers"), Variant=w1399) -> (data=w1394:u16[], error out=w1393:errorcluster)
        n403 = call "DisplayValuesFromPLC.vi"("PLC Data"=w1381, "error in"=w1393, "Input Registers"=w1394) -> ("error out"=w1392:errorcluster, "PLC Data Out"=w1391:T3)  [unwired: 7 in]
        n404 = call "DisplayValuesFromPLC_LDO.vi"("error in"=w1392, "PLC Data"=w1391) -> ("error out"=w1387:errorcluster, "PLC Data Out"=w1389:T3)  [unwired: 8 in]
        n405 = call "FVIR Button Disable.vi"("UI Refs"=w1390, "error in (no error)"=w1387, "PLC Data In"=w1389, "Queue in"=w1397) -> ("error out"=w1386:errorcluster, "PLC Data Out"=w1388:T3, "Queue out"=w1396:refnum<queue>)  [unwired: 5 in]
        n406 = call "LDO Button Disable.vi"("UI Refs"=w1390, "error in (no error)"=w1386, "PLC Data In"=w1388, "Queue in"=w1396) -> ("error out"=w1383:errorcluster, "PLC Data Out"=w1379:T3, "dup Message Queue"=w1384:refnum<queue>)  [unwired: 5 in]
        n407 = call-poly "Enqueue Message.vi"("error in (no error)"=w1383, "Message"="DisplayAllData", "Message Queue"=w1384) -> ("error out"=w1382:errorcluster)  [unwired: 7 in, 1 out]
        n408 = Bundle By Name(cluster=w1380, "PLC Data Out"=w1379) -> (w1378:T2)
      }
      frame "DisplayValuesFromAlicat_LDO" {
        n409 = Variant To Data(error in=w1411, type=T7 {"Data Cluster"={"Absolute Pressure"=0.0, "Gauge/Diff. Pressure"=0.0, "Barometric Pressure"=0.0, "Temperature"=0.0, "Volumetric Flow"=0.0, "Mass Flow"=0.0, "Setpoint"=0.0, "Valve Drive"=0.0, "Totalizer"=0.0, "[hr]"=0.0, "[min]"=0.0, "[sec]"=0.0, "Totalizer Average Flow"=0.0, "Totalizer Peak Flow"=0.0, "Gas selected"=""}, "Units of Measure Input"={"Abs. Pressure"="", "Gauge/Diff. Press."="", "Barometric Press."="", "Temperature"="", "Volume"="", "Mass"="", "Setpoint"="", "Valve Drive"="", "Totalizer"="", "Tot. Timer"="", "Tot. Avg. Flow"="", "Tot. Peak Flow"=""}, "Header Array"=[]} ("Gas Data"), Variant=w1410) -> (data=w1402:T7, error out=w1407:errorcluster)
        n410 = Bundle By Name(cluster=w1404, "Gas Data"=w1402) -> (w1403:T2)
        n411 = call-poly "Enqueue Message.vi"("error in (no error)"=w1407, "Message"="DisplayAllData", "Message Queue"=w1408) -> ("error out"=w1406:errorcluster)  [unwired: 7 in, 1 out]
      }
      frame "DisplayValuesFromInficon" {
        w1423 = T10 {"Gross Heating Value, Vol (Real, Dry)"=0.0, "Nitrogen Component Normalized Mole % (Dry)"=0.0, "Methane Component Normalized Mole % (Dry)"=0.0, "Carbon Dioxide Component Normalized Mole % (Dry)"=0.0, "Ethane Component Normalized Mole % (Dry)"=0.0, "Propane Component Normalized Mole % (Dry)"=0.0, "i-Pentane Component Normalized Mole % (Dry)"=0.0, "i-Butane Component Normalized Mole % (Dry)"=0.0, "n-Butane Component Normalized Mole % (Dry)"=0.0, "n-Pentane Component Normalized Mole % (Dry)"=0.0, "Hexane Component Normalized Mole % (Dry)"=0.0, "Heptane Component Normalized Mole % (Dry)"=0.0, "Gross Wobbe Index, Real(Dry)"=0.0, "Relative Density, Real(Dry)"=0.0, "Propylene Component Normalized Mole % (Dry)"=0.0, "C4 Olefins Component Normalized Mole % (Dry)"=0.0, "Water Component Normalized Mole % (Dry)"=0.0}  # Inficon Data Input
        n412 = Variant To Data(error in=w1424, type=w1423, Variant=w1422) -> (data=w1415:T10, error out=w1420:errorcluster)
        n413 = Bundle By Name(cluster=w1417, "Inficon Data Input"=w1415) -> (w1416:T2)
        n414 = call-poly "Enqueue Message.vi"("error in (no error)"=w1420, "Message"="DisplayAllData", "Message Queue"=w1418) -> ("error out"=w1419:errorcluster)  [unwired: 7 in, 1 out]
      }
      frame "DisplayValuesFromUltramat" {
        n415 = Variant To Data(error in=w1437, type=string[][] [], Variant=w1436) -> (data=w1428:string[][], error out=w1434:errorcluster)
        n416 = Bundle By Name(cluster=w1431, "Ultramat 23"=w1428) -> (w1430:T2)
        n417 = call-poly "Enqueue Message.vi"("error in (no error)"=w1434, "Message"="DisplayAllData", "Message Queue"=w1432) -> ("error out"=w1433:errorcluster)  [unwired: 7 in, 1 out]
      }
      frame "CheckBeforeWriteDataLDO" {
        n418 = Unbundle By Name(w1441) -> ("PLC Data Out"=w1440:T3)
        n419 = call-poly "Enqueue Message.vi"("error in (no error)"=w1445, "Message Data"=w1440, "Message"="CheckBeforeWriteDataLDO", "Message Queue"=w1443) -> ("error out"=w1444:errorcluster)  [unwired: 6 in, 1 out]
      }
      frame "CheckBeforeWriteDataFVIR" {
        n420 = Unbundle By Name(w1450) -> ("PLC Data Out"=w1449:T3)
        n421 = call-poly "Enqueue Message.vi"("error in (no error)"=w1454, "Message Data"=w1449, "Message"="CheckBeforeWriteDataFVIR", "Message Queue"=w1452) -> ("error out"=w1453:errorcluster)  [unwired: 6 in, 1 out]
      }
      frame "Error" {
        # "Error - Display an error dialog. This message is sent by the \"Error Handler\" VIs at the end of other loops in this application."
        n422 = Variant To Data(error in=w1461, type=errorcluster {"status"=FALSE, "code"=0, "source"=""} ("error constant"), Variant=w1464) -> (data=w1462:errorcluster, error out=w1465:errorcluster)
        n423 = call <vilib>:"Simple Error Handler.vi"("error in (no error)"=w1462) -> ()  [unwired: 4 in, 5 out]
        n424 = Merge Errors(w1465) -> (w1463:errorcluster)
      }
      frame "Exit" {
        w1471 = TRUE ("Priority Message? (F)")
        w1469 = "Exit" ("Message")
        # "Popup an error dialog if 'Exit' was called as a result of an error."
        # "Stop the VI"
        # "Exit - Send Exit messages to the Acquisition and Logging loops, and fire the user event to stop the Event Handling Loop."
        n425 = Variant To Data(type=errorcluster {"status"=FALSE, "code"=0, "source"=""} ("error constant"), Variant=w1489) -> (data=w1488:errorcluster)  [unwired: 1 in, 1 out]
        n426 = call <vilib>:"Simple Error Handler.vi"("error in (no error)"=w1488) -> ()  [unwired: 4 in, 5 out]
        n427 = call-poly "Enqueue Message.vi"("Priority Message? (F)"=w1471, "error in (no error)"=w1481, "Message"=w1469, "Message Queue"=w1487) -> ("error out"=w1486:errorcluster)  [unwired: 6 in, 1 out]
        n428 = call-poly "Enqueue Message.vi"("Priority Message? (F)"=w1471, "error in (no error)"=w1486, "Message"=w1469, "Message Queue"=w1485) -> ("error out"=w1484:errorcluster)  [unwired: 6 in, 1 out]
        n429 = call-poly "Enqueue Message.vi"("Priority Message? (F)"=w1471, "error in (no error)"=w1484, "Message"=w1469, "Message Queue"=w1483) -> ("error out"=w1480:errorcluster)  [unwired: 6 in, 1 out]
        n430 = call-poly "Enqueue Message.vi"("Priority Message? (F)"=w1471, "error in (no error)"=w1480, "Message"=w1469, "Message Queue"=w1479) -> ("error out"=w1478:errorcluster)  [unwired: 6 in, 1 out]
        n431 = call-poly "Enqueue Message.vi"("Priority Message? (F)"=w1471, "error in (no error)"=w1478, "Message"=w1469, "Message Queue"=w1477) -> ("error out"=w1475:errorcluster)  [unwired: 6 in, 1 out]
        n432 = call-poly "Enqueue Message.vi"("Priority Message? (F)"=w1471, "error in (no error)"=w1475, "Message"=w1469, "Message Queue"=w1474) -> ("error out"=w1473:errorcluster)  [unwired: 6 in, 1 out]
        n433 = call-poly "Enqueue Message.vi"("Priority Message? (F)"=w1471, "error in (no error)"=w1473, "Message"=w1469, "Message Queue"=w1470) -> ("error out"=w1472:errorcluster)  [unwired: 6 in, 1 out]
        n434 = call "Fire User Event - Stop.vi"("error in (no error)"=w1472, "User Event - Stop"=w1493) -> ("error out"=w1492:errorcluster)  [unwired: 9 in]
      }
      frame "---Copy This Frame---" {
        # "Duplicate this frame when creating new messages.  Change this comment in the duplicated frame to describe this message."
        n435 = Merge Errors(w1500) -> (w1499:errorcluster)
      }
      frame Default {
        # "'Default' case only runs if there is a message that isn't defined in any of the other cases.  Output a programming error."
        n436 = xnode "Error Ring"("parameter 0"=w1505) -> ("error out"=w1504:errorcluster)
      }
    }
    n437 = case shown="True" "Debug" {
      tunnel: w371 -> [w397 w400]
      tunnel: w370 -> [_ w399]
      tunnel: [w397 w398] -> w369
      frame False {
      }
      frame True {
        n438 = Build Array (concatenate)(w400, w399) -> (w398:string[])
        "Message Loop" <- w398
      }
    }
    n439 = call "Error Handler - Message Handling Loop.vi"("error in (no error)"=w387, "Message Queue"=w386) -> ("dup error in"=w388:errorcluster)  [unwired: 8 in, 1 out]
    "UI Message Loop" <- w374
  }
  n440 = Unregister For Events(event registration refnum=w33, error in=w36) -> (error out=w34:errorcluster)
  n441 = Release Queue(queue=w20, error in (no error)=w37) -> (error out=w21:errorcluster)  [unwired: 1 in, 2 out]
  n442 = Merge Errors(w34, w21, w24, w23, w22, w19, w10, w9, w8) -> (w31:errorcluster)
  n443 = call "Destroy User Event - Stop.vi"("error in (no error)"=w31, "User Event - Stop"=w27) -> ("error out"=w30:errorcluster)  [unwired: 9 in]
  n444 = disable-structure shown="Default" {
    disable-tunnel: w30 -> [_ _]
    frame condition #0 (active) {
    }
    frame condition #1 {
      # "Call Quit LabVIEW if running as a built application."
      n445 = Quit LabVIEW() -> ()  [unwired: 1 in]
    }
  }
